vi "Position_TOTAL_R13.vi"(5 "Distance Between \nCameras  (*unit)":sgl=2.6) -> (0 "Valid Beacon Sets":bool[](array[boolean])=[TRUE, TRUE, TRUE, TRUE, TRUE], 12 "dX, dY\nLeft Cam":cluster{"X":sgl[], "Y":sgl[]}={"X"=[-3.0932024, -2.0237627, -0.92593014, 0.110565156, 1.1772758], "Y"=[9.218185, 9.218186, 9.218185, 9.218184, 9.218185]}, 13 "Position Valid":bool=TRUE, 14 "Left Camera Real Coordinates":cluster{"X":sgl, "Y":sgl}={"X"=9.218185, "Y"=3.507011}, 16 "dX, dY\nRight Cam":cluster{"X":sgl[], "Y":sgl[]}={"X"=[-5.4051104, -4.335671, -3.237838, -2.2013428, -1.1346322], "Y"=[8.902709, 8.902709, 8.902709, 8.902708, 8.902709]}, 17 "Distance to Each Beacon":cluster{" Right Cam":sgl[], " Left Cam":sgl[]}={" Right Cam"=[10.394308, 9.916446, 9.480992, 9.198957, 8.942072], " Left Cam"=[9.7002945, 9.453048, 9.272804, 9.247818, 9.26041]}, 18 "Robot Coordinates":cluster{"X":sgl, "Y":sgl}={"X"=9.060447, "Y"=4.662965}, 19 "Orietnation\n(current)":sgl=-7.7704344 format="%#_13g")   [LabVIEW 2015]
uses:
  <vilib>/Analysis/coordinate.llb/2D Cartesian Coordinate Rotation (Array).vi
  <vilib>/myRIO/Common/Instrument Driver Framework/myRIO v1.0/DIO/vis/myRIO v1.0 Close DIO.vi
  <vilib>/myRIO/Common/Instrument Driver Framework/myRIO v1.0/DIO/vis/myRIO v1.0 Unreserve DIO.vi
  <vilib>/myRIO/Common/Instrument Driver Framework/myRIO v1.0/DIO/vis/myRIO v1.0 Build MUX Configuration DIO.vi
  <vilib>/myRIO/Common/Instrument Driver Framework/myRIO v1.0/Resource Manager/vis/myRIO v1.0 Unreserve Channel List.vi
  <vilib>/myRIO/Common/Instrument Driver Framework/myRIO v1.0/Resource Manager/vis/myRIO v1.0 Create Configuration List.vi
  <vilib>/myRIO/Common/Instrument Driver Framework/myRIO v1.0/Resource Manager/vis/myRIO v1.0 Unreserve Channel.vi
  <vilib>/myRIO/Common/Instrument Driver Framework/myRIO v1.0/Resource Manager/vis/myRIO v1.0 Build Mutex Name.vi
  <vilib>/Instr/_visa.llb/VISA Configure Serial Port (Instr).vi
  <vilib>/myRIO/Common/Instrument Driver Framework/myRIO v1.0/DIO/vis/myRIO v1.0 Shutdown DIO.vi
  <vilib>/Utility/error.llb/Error Cluster From Error Code.vi
  <vilib>/myRIO/Common/Instrument Driver Framework/myRIO v1.0/Resource Manager/vis/myRIO v1.0 Configure IO.vi
  <vilib>/myRIO/Common/Instrument Driver Framework/Utilities/vis/Configuration Manager.vi
  <vilib>/myRIO/Common/Instrument Driver Framework/Utilities/vis/IO Manager.vi
  <vilib>/myRIO/Common/Instrument Driver Framework/myRIO v1.0/myRIO v1.0 Close.vi
  <vilib>/Analysis/NI_AALPro.lvlib
  <vilib>/myRIO/Instrument Drivers/Onboard IO/DIO/DIO.lvlib
panel:
  in  "Position Calc\nTimer":u32=50 caption="Position Calc Timer"
  in  "Max Dual\nBad Count":i32=10
  in  "Fetch Input\n(mSec)":u32=20 caption="Update Camera Input\n(mSec)"
  out "Right Data\nInput Flag\n- Internal":bool=TRUE
  in  "Position Calc\nReady":bool
  out "This Servo \nAngle - Right":sgl=88.125
  in  "Beacon Angles -R":sgl[](array[numeric])
  in  "Beacon Angles - L":sgl[](array[numeric])
  in  "Valid Angles -R":bool[](array[boolean])=[TRUE, TRUE, TRUE, TRUE, TRUE]
  in  "Valid Angles - L":bool[](array[boolean])=[TRUE, TRUE, TRUE, TRUE, TRUE]
  out "Left Data\nInput Flag\n- Internal":bool=TRUE
  in  "Check Shared Var Timer":u32=50 caption="Main Loop\n Timer (ms)"
  out "Left_Flag 2":bool
  out "Right_Flag 2":bool
  out "Beacons Found\n- Left (Bool Array) 2":bool[](array[boolean])=[TRUE, TRUE, TRUE, TRUE, TRUE]
  out "LEFT Beacon Coord - X px (IN) 2":sgl[](array[numeric])=[180.1461, 249.37689, 322.34314, 385.45602, 466.0847]
  out "LEFT Beacon Position - Y px (IN) 2":sgl[](array[numeric])=[301.75427, 303.58112, 297.41064, 306.23984, 296.68478]
  out "This Servo \nAngle - Left":sgl=88.125
  out "dT - Logic Loop":u32=134
  in  "Compliance Slope":u8=128
  in  "Max Search\n- Reactive Search Timeout":i32=10
  in  "Max Smart \nSearch Attempts":i32=50
  out "Search Count - R":u16
  out "Last Known\nTracking Position - R":u16=352
  out "Recovery Search Count R":i32
  out "Current Step - R":i8=9
  out "Response\nInduced - R":bool
  out "Response\nInduced - L":bool
  out "Pll Induced":bool
  out "Recovery Search Count L":i32
  out "deltaMoveServo\n- R":i16=52
  out "Move Respond - R":bool
  out "Move Respond - L":bool
  in  "Middle Beacon Coordinates":cluster{"X":sgl, "Y":sgl}={"X"=0.0, "Y"=2.5}
  out "Last Position":cluster{"X":sgl, "Y":sgl}
  out "Last Orientation":sgl
  in  "Distance\nBetween Beacons \n- Tolerance":sgl=0.35 format="%#_13g"
  in  "Distance\nBetween Beacons":sgl=1.0 format="%#_13g"
  out "atan2(y,x)":sgl
  out "dT":dbl
  in  "Orientation (-2) \nWeight":sgl=0.083333336 format="%#_13g"
  in  "Orientation (-1) \nWeight":sgl=0.16666667 format="%#_13g"
  in  "New Orientation \nThreshold":sgl=10.0
  out "Position Valid\nHistory":bool[](array[boolean])
  out "Orientation\nHistory":sgl[](array[numeric])
  out "Robot Coordinates\nHistory":cluster{sgl, sgl}[](array[cluster])
  in  "New Position \nThreshold":sgl=1.0
  in  "position(-2) weight":sgl=0.15 format="%#_13g"
  in  "position(-1) weight":sgl=0.35 format="%#_13g"
  out "Orientation Avgd":sgl
  in  "History Size":u8=10
  in  "Max Y (arena)":sgl=15.0
  in  "Max X (arena)":sgl=28.0
  in  "New Position\nWeight":sgl=0.5 format="%#_13g"
  in  "New Orientation\nWeight":sgl=0.75 format="%#_13g"
  in  "Max Std Dev (3)":sgl=0.2 format="%#_13g"
  in  "Max Std Dev (4)":sgl=0.2 format="%#_13g"
  out "Post Filtering\n- Valid Beacons":bool[](array[boolean])
  in  "New Pos\nThreshold (*unit)\nfilterd UNUSED":sgl=0.2
  out "Robot Coordinates - Avgd":cluster{"X":sgl, "Y":sgl}={"X"=9.06069, "Y"=4.637566}
  out "Real Position in Course 2":cluster{"X":dbl[], "Y":dbl[]}(graph)={"X"=[0.0, 0.0, 0.0, 0.0, 0.0, 9.060689926147461], "Y"=[0.5, 1.54, 2.58, 3.58, 4.58, 4.637566089630127]}
  out "Position \nLock Status":bool=TRUE
  in  "Max delta Angle":i32=1000
  out "Array 2":i16[](array[numeric])=[6, 1, 2, 14, 12]
  out "Right Camera Real Coordinate":cluster{"X":sgl, "Y":sgl}={"X"=8.902709, "Y"=5.8189187}
  in  "Start Search\nThreshold\n (x Wait Thres)":i32=5
  in  "Right Manual\nAngle":sgl=90.0
  in  "Left Manual\nAngle":sgl=90.0
  in  "MANUAL SERVO \nCONTROL ENABLE":bool
  out "deltaMoveServo\n- L":i16=52
  out "Last Known\nTracking Position - L":u16=352
  out "Search Count - L":u16
  in  "Search Step Size\n(deg)":sgl=10.0 format="%#_13g"
  out "Beacons Found\n- Right (Bool Array)":bool[](array[boolean])=[TRUE, TRUE, TRUE, TRUE, TRUE]
  out "RIGHT Beacon Position - Y px (IN)":sgl[](array[numeric])=[286.47595, 290.1055, 289.42014, 306.0349, 296.24573]
  out "RIGHT Beacon Coord - X px (IN)":sgl[](array[numeric])=[198.15767, 257.3629, 323.06607, 420.0157, 463.01376]
  in  "Right Servo\nID":string="\u0001"
  in  "Servo Comm\nWait Time - (ms)":i32
  in  "Left Servo\nID":string="\u0000"
  out "dT - Comm Loop":u32=134
  in  "Servo Comm\nLoop Time (ms)":i32=10
  in  "close comms":bool
  in  "Max Read\nTx Attempts":u8=3
  in  "Max Write\nTx Attempts":u8=3
  out "Current R (10bit)":u16=709
  out "Servo Moving - R":bool
  out "Servo Moving - L":bool
  out "Current L (10bit)":u16=352
  in  "SERVO ENABLE":bool=TRUE
  out "Move Servo - L":bool
  out "Move Servo - R":bool
  in  "Servo Goal Position\n - Right":u16=707
  in  "Move Servo\nThreshold (deg)":sgl=2.0 format="%#_13g"
  out "Current Step - L":i8=9
  in  "Angles Valid - L":bool=TRUE
  out "Wait Cycle Count - L":i32
  out "Wait Count - R":i32
  in  "Angles Valid - R":bool=TRUE
  in  "Wait Count\nFactor":i32=15
  in  "Servo Algorithm\nCycle Time(ms)":i32=50
  out "Direction - L":bool
  out "Direction - R":bool=TRUE
  in  "Servo Goal Position\n - Left":u16=353
  in  "Middle Beacon\nAngle - Left":sgl=87.88366
  in  "Current Angle\n - Left (internal)":sgl=88.125
  in  "Middle Beacon\nAngle - Right":sgl=102.09343
  in  "Current Angle\n - Right (internal)":sgl=102.71484
  in  "stop":bool
  in  "Num of Beacons (Total)":i8=5
  out "Angle to Pixel Ratios":T1={"Angle to Pixel\nRatio - Horizontal"=0.090625, "Angle to Pixel\nRatio - Vertical"=0.09375} {"Angle to Pixel\nRatio - Vertical" format="%#_13g"; "Angle to Pixel\nRatio - Horizontal" format="%#_13g"}
  in  "Cam AOV Vertical (deg)":sgl=45.0
  in  "Cam AOV Horizontal (deg)":sgl=58.0
  in  "Image Height (px)":sgl=480.0
  in  "Image Width (px)":sgl=640.0
  out "Beacon Coordinates - Left Image":T2={"Beacon Position - X px"=[-75.0, 0.0, 102.0], "Beacon Position - Y px"=[133.0, 0.0, 40.0]}
  out "Beacon Coordinates - Right Image":T2
  out "Distance to LBF":sgl[](array[numeric])=[0.024284193, 0.015691843, 0.008273765, 0.028971607, 0.03291407]
  out "Local Coordinates - Calculated":cluster{sgl[], sgl[]}(graph)={[-1.8217448, -0.75672, 0.3300292, 1.3598052, 2.408354], [9.527695, 9.422711, 9.26693, 9.147298, 8.941757]}
  out "Local Coordinates - Adjusted":cluster{sgl[], sgl[]}(graph)={[-1.8184614, -0.75884163, 0.32891047, 1.3558882, 2.4128041], [9.551756, 9.407164, 9.258732, 9.118592, 8.974369]}
  out "Normalized Beacons\nCoordinates Relative\nto Robot\n- Local":cluster{"X":sgl[], "Y":sgl[]}={"X"=[-1.8184614, -0.75884163, 0.32891047, 1.3558882, 2.4128041], "Y"=[9.551756, 9.407164, 9.258732, 9.118592, 8.974369]}
  out "Local Coordinates - Rotated":cluster{dbl[], dbl[]}(graph)={[2.311907982053154, -3.093202399055953, -2.02376281856378, -0.9259301209089894, 0.11056515513330578, 1.1772757583589313], [0.3154767124369396, 9.218185381048452, 9.218185941536527, 9.218185875284743, 9.218184915244796, 9.218185579154817]}
  out "All Object Coordinates \n- Local - Rotated":cluster{"X":sgl[], "Y":sgl[]}={"X"=[2.311908, -3.0932024, -2.0237627, -0.92593014, 0.110565156, 1.1772758], "Y"=[0.31547672, 9.218185, 9.218186, 9.218185, 9.218184, 9.218185]}
  out "Local Coordinates - Normalized":cluster{sgl[], dbl[]}(graph)={[2.3333333, -1.8184614, -0.75884163, 0.32891047, 1.3558882, 2.4128041], [0.0, 9.551755905151367, 9.407163619995117, 9.258731842041016, 9.118592262268066, 8.974369049072266]}
  in  "Max Std Dev (5)":sgl=0.2 format="%#_13g"
  out "All Object Coordinates \n- Local":cluster{"X":sgl[], "Y":sgl[]}={"X"=[2.3333333, -1.8184614, -0.75884163, 0.32891047, 1.3558882, 2.4128041], "Y"=[0.0, 9.551756, 9.407164, 9.258732, 9.118592, 8.974369]}
  out "LOCAL\nBeacon Coordinates\nRelative to Robot":cluster{"dX_beacon":sgl[], "dY_beacon":sgl[]}={"dX_beacon"=[-1.8217448, -0.75672, 0.3300292, 1.3598052, 2.408354], "dY_beacon"=[9.527695, 9.422711, 9.26693, 9.147298, 8.941757]}
  out "dA2":sgl=15.074211 format="%#_13g"
  out "All Same\nDirection":bool=TRUE
  out "Valid Data\nSets":bool[](array[boolean])=[TRUE, TRUE, TRUE, TRUE, TRUE]
  in  "Distance Threshold\nRef Triangles (*unit)":sgl=20.0
  in  "Real Beacon\n - Coordinates":cluster{"X":dbl[], "Y":dbl[]}={"X"=[0.0, 0.0, 0.0, 0.0, 0.0, 0.0], "Y"=[0.5, 1.5, 2.5, 3.5, 4.5, 0.0]}
  # "POSITION CALCULATION VARIABLES"
  # "OUTPUT VALUES"
  # "CONFIG VALUES"
  # "FILTER CONFIG VALUES"
  # "FEEDBACK INPUT VALUES"
  # "INPUT VALUES"
  # "INTERMEDIATE VALUES"
  # "IMAGE TO ANGLE VARIABLES"
  # "VISION PROCESSEING INPUTS"
  # "Use moving average for previous orientation thresholds"
  # "INPUTS"
  # "CONFIG"
  # "OUTPUT VALUES"
  # "*********************"
  # "unfiltered"
  # "NEW FILTER VALS"
  # "Inter Beacon Distance Filtering"
  # "SERVO CONTROL VARIABLES"
  # "SERVO CONTROL VARIABLES"
  # "CONFIG"
  # "SHARED VARIABLE INPUTS"
  # "LOCAL VARIABLE INPUTS"
  # "INTERNRAL VARIABLES"
  # "SEARCH ROUTINE VARIABLES"
  # "MISC"
  # "SERVO IDs"
  # "CONTROL DELAYS"
  # "COMM LOOP DELAY"
  # "COMM PROTOCOL"
  # "1 Search Cycle is Certain\nNumber of Wait Cycles"
  # "Servo Enable must be false**"
  # "Make function of distance^^"
  # "**** only left side starts search\nat previously known good angle"
  # "change to only use\nthis max delta angle\nwhen enabled"
  # "NOTE: Must be 1 bigger than amount of beacons"
  # "NOTE: Must be 1 bigger than amount of beacons"
types:
  T1 = cluster{"Angle to Pixel\nRatio - Horizontal":sgl, "Angle to Pixel\nRatio - Vertical":sgl}
  T2 = cluster{"Beacon Position - X px":sgl[], "Beacon Position - Y px":sgl[]}
  T3 = cluster{"Array of Double":dbl[], "Array of Double":dbl[]}
  T4 = typedef "DIO.lvlib/DIO Reference.ctl" = cluster{"myRIO Reference":T5, "DIO Channels List":T9}
  T5 = typedef "myRIO Generic Hardware Reference.ctl" = cluster{"myRIO Model":T6, "myRIO Hardware Reference":T7}
  T6 = typedef "Hardware Version Enum.ctl" = enum16{"Unknown", "myRIO-1900", "myRIO-1950", "roboRIO"}
  T7 = typedef "myRIO v1.0 Reference.ctl" = cluster{"Generic FPGA Reference":T8, "Allow multiple opens":bool}
  T8 = typedef "Generic FPGA Reference.ctl" = refnum<k20>
  T9 = typedef "DIO Channels List.ctl" = T10[]
  T10 = typedef "DIO Channels Enum.ctl" = enum16{"Not Connected", "C/DIO0", "C/DIO1", "C/DIO2", "C/DIO3", "C/DIO4", "C/DIO5", "C/DIO6", "C/DIO7", "A/DIO0", "A/DIO1", "A/DIO2", "A/DIO3", "A/DIO4", "A/DIO5", "A/DIO6", "A/DIO7", "A/DIO8", "A/DIO9", "A/DIO10", "A/DIO11", "A/DIO12", "A/DIO13", "A/DIO14", "A/DIO15", "B/DIO0", "B/DIO1", "B/DIO2", "B/DIO3", "B/DIO4", "B/DIO5", "B/DIO6", "B/DIO7", "B/DIO8", "B/DIO9", "B/DIO10", "B/DIO11", "B/DIO12", "B/DIO13", "B/DIO14", "B/DIO15", "LED0", "LED1", "LED2", "LED3", "Button0", "DIO/DIO0", "DIO/DIO1", "DIO/DIO2", "DIO/DIO3", "DIO/DIO4", "DIO/DIO5", "DIO/DIO6", "DIO/DIO7", "DIO/DIO8", "DIO/DIO9", "SPI/CS0", "SPI/CS1", "SPI/CS2", "SPI/CS3", "LED RADIO (Green)", "LED RADIO (Red)", "LED COMM (Green)", "LED COMM (Red)", "LED MODE (Green)", "LED MODE (Red)"}
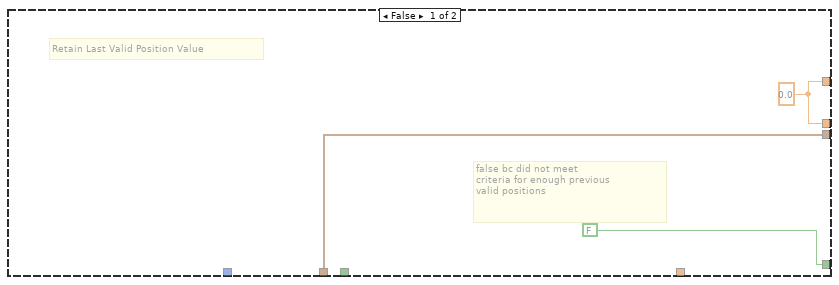
[diagram p6: hidden frame]
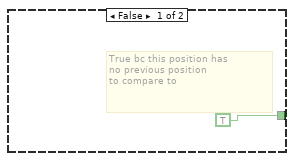
[diagram p7: hidden frame]
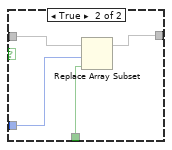
[diagram p9: hidden frame]
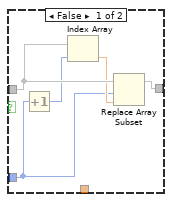
[diagram p10: hidden frame]
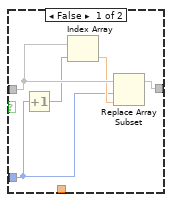
[diagram p11: hidden frame]
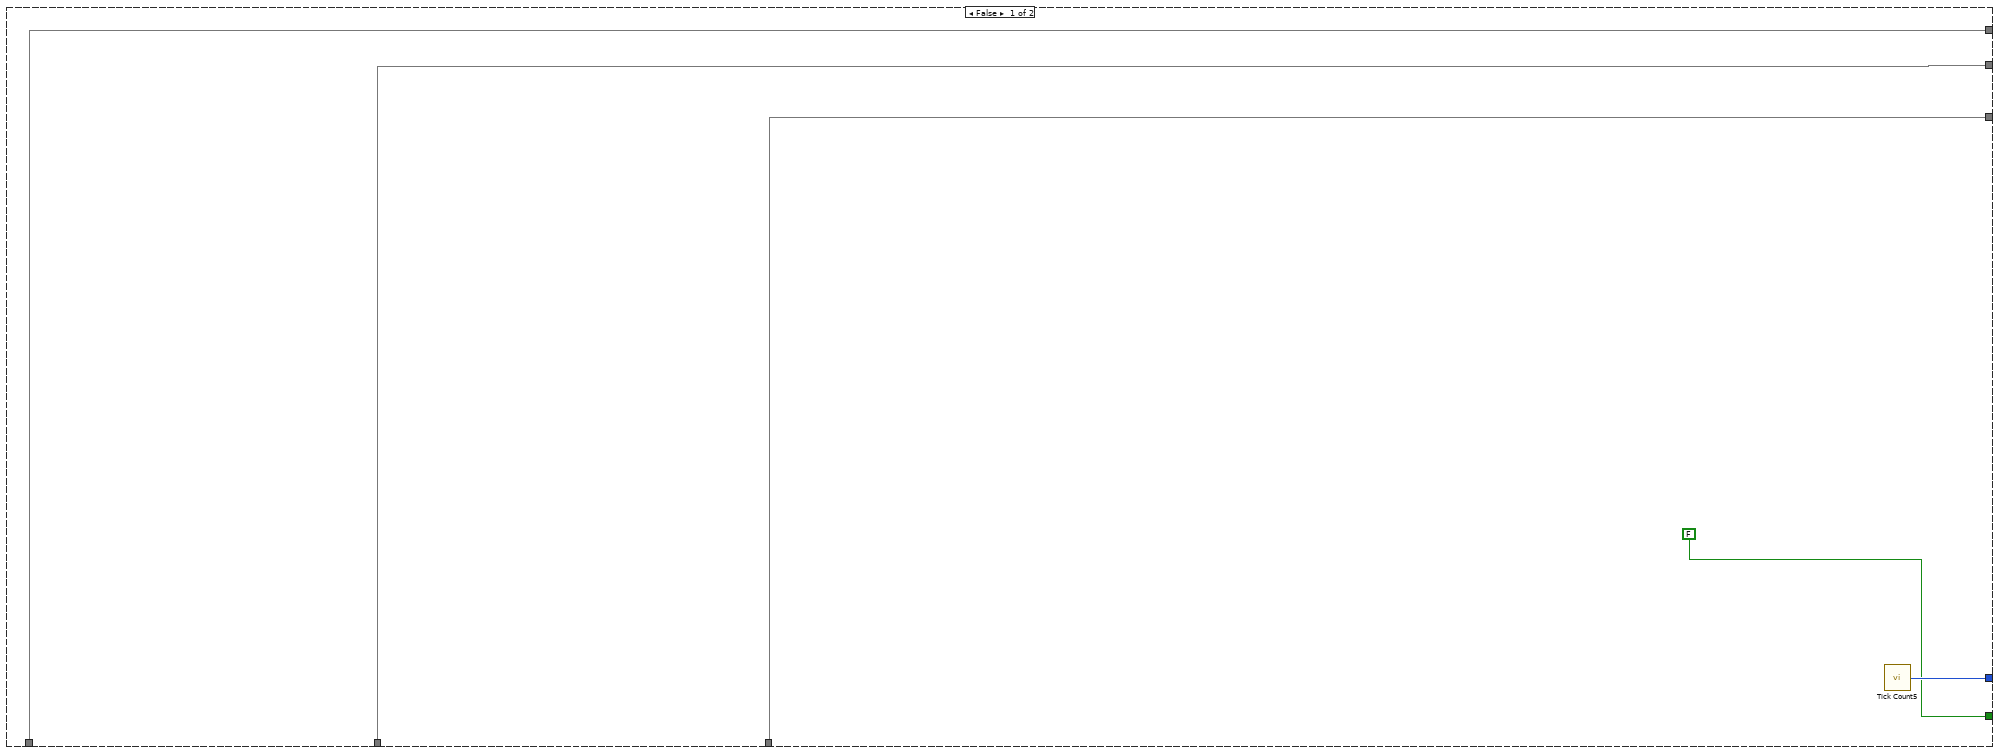
[diagram p14: hidden frame]
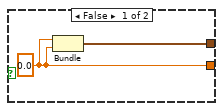
[diagram p16: hidden frame]
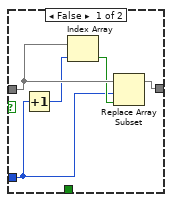
[diagram p17: hidden frame]
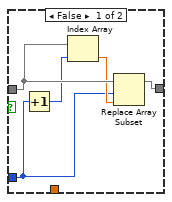
[diagram p18: hidden frame]
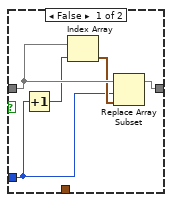
[diagram p19: hidden frame]
diagram:
  w4 = FALSE
  w1 = FALSE
  w23 = sgl 0.0
  w15 = u16 35
  w16 = u16 512
  # "Completel Search Mode"
  # "Read Inputs when Available"
  # "# of Physical Beacons"
  # "Right Data Internal Falg"
  # "Left Data Internal Falg"
  # "Start at (or around)\nMax Smart Search\nso system will\nimmediately begin to search"
  # "Recovery Search -5"
  # "Recovery Search - L"
  # "Search Count - R"
  # "Direction - R"
  # "Direction - L"
  # "Wait Cycle Count"
  # "Search Cycle Count - R"
  # "Last Known Track\nAngle - R"
  # "Move Respond - R"
  # "Move Respond - L"
  # "Move Respond - R"
  # "Move Respond - L"
  # "Wait Cycle Count"
  # "Last Known Track\nAngle"
  # "Search Count - L"
  # "delta Move Angle - R\n(Sum)"
  # "delta Move Angle - L\n(Sum)"
  # "delta Move Angle - R"
  # "delta Move Angle - L"
  # "Last Known Track\nAngle - L"
  # "Initialize Shift Arrays"
  # "Robot Position (cluster)\nShift Array"
  # "Robot Position (cluster)\nShift Array"
  # "Position Valid Shift Array"
  # "Orientation Shift Array"
  # "Position Valid Shift Array"
  # "Orientation Shift Array"
  # "***********************************"
  # "Search Cycle Count - L"
  # "Servo Communication (to Servo- UART))"
  # "Wait Cycle Counter - R"
  # "Internal Local Variables"
  # "Servo Control Logic"
  # "Wait Cycle Counter - L"
  # "Local Variables"
  # "Images to Robot Position Calculation Process"
  # "SERVO MOTOR CONTROL"
  # "SERVO MOTOR CONTROL"
  n1 = Divide(x="Cam AOV Horizontal (deg)", y="Image Width (px)") -> (x/y=w9:sgl)
  n2 = Divide(x="Cam AOV Vertical (deg)", y="Image Height (px)") -> (x/y=w10:sgl)
  n3 = Bundle(w9, w10) -> (w3:cluster{sgl, sgl})  [unwired: 1 in]
  "Angle to Pixel Ratios" <- w3
  n4 = disable-structure shown="Disabled" {
    frame Disabled {
      # "Always Read Incoming Flags & Store"
      n5 = while {
        tunnel: "Check Shared Var Timer" -> [w40]
        stop <- FALSE stop-if-true
        n6 = shared-variable "myRIO-1900\\Lib1.lvlib\\RIGHT_FLAG"() -> (→"Right_Flag 2":bool)  [unwired: 1 in, 1 out]
        n7 = shared-variable "myRIO-1900\\Lib1.lvlib\\Left_Flag"() -> (→"Left_Flag 2":bool)  [unwired: 1 in, 1 out]
        n8 = call "Wait8"("Count(mSec)"=w40) -> ()  [unwired: 1 out]
      }
    }
    frame Enabled {
    }
  }
  n9 = while {
    shift-right: [w48] -> _
    shift-left: w4 -> [w54]
    shift-right: [w47] -> _
    shift-left: w4 -> [w52]
    tunnel: w3 -> [w50]
    tunnel: "Num of Beacons (Total)" -> [w51]
    stop <- FALSE stop-if-true
    # "Wait for Both Internal Flags"
    n10 = call "Wait6"("Count(mSec)"="Fetch Input\n(mSec)") -> ()  [unwired: 1 out]
    n11 = shared-variable "RT myRIO Target - Overlord\\Localization_Variables_r0.lvlib\\RIGHT_FLAG"() -> (w44:bool)  [unwired: 1 in, 1 out]
    n12 = shared-variable "RT myRIO Target - Overlord\\Localization_Variables_r0.lvlib\\Left_Flag"() -> (w45:bool)  [unwired: 1 in, 1 out]
    n13 = case shown="True" w44 {
      tunnel: w51 -> [_ w68]
      tunnel: w50 -> [_ w66]
      tunnel: [w55 TRUE] -> w43
      tunnel: w52 -> [w55 _]
      frame False {
        # "Don't Update Servo Position\nbc we're waiting on new Data to\ncome in and the servo position\nwas set at the previous set of data"
      }
      frame True {
        # "Store Values"
        # "Raise Internal Flag"
        # "If New Data Available"
        # "From Shift Reg"
        # "Perforrm Indivudual Angle Calculation"
        # "Pull Down Individual Flag"
        n14 = shared-variable "RT myRIO Target - Overlord\\Localization_Variables_r0.lvlib\\RIGHT_BEACON_X_array"() -> (w60:dbl[])  [unwired: 1 in, 1 out]
        "RIGHT Beacon Coord - X px (IN)" <- w60
        n15 = shared-variable "RT myRIO Target - Overlord\\Localization_Variables_r0.lvlib\\RIGHT_BEACON_Y_array"() -> (w59:dbl[])  [unwired: 1 in, 1 out]
        "RIGHT Beacon Position - Y px (IN)" <- w59
        n16 = shared-variable "RT myRIO Target - Overlord\\Localization_Variables_r0.lvlib\\RIGHT_BEACON_BOOL_array"() -> (w58:bool[])  [unwired: 1 in, 1 out]
        "Beacons Found\n- Right (Bool Array)" <- w58
        n17 = Bundle("Array of Double"=w60, "Array of Double"=w59) -> (w57:T3)  [unwired: 1 in]
        "Beacon Coordinates - Right Image" <- w57
        n18 = shared-variable "RT myRIO Target - Overlord\\Localization_Variables_r0.lvlib\\Right Servo Angle_Image"() -> (w56:dbl)  [unwired: 1 in, 1 out]
        "This Servo \nAngle - Right" <- w56
        n19 = shared-variable "RT myRIO Target - Overlord\\Localization_Variables_r0.lvlib\\RIGHT_FLAG"(FALSE) -> ()  [unwired: 1 in, 1 out]
        n20 = feedback #1() -> (w70:sgl[])  [unwired: 1 in]
        n21 = feedback #2() -> (w69:bool[])  [unwired: 1 in]
        n22 = call "Angle Calc_Individual Process R2.vi"("Angle to Pixel Ratios"=w66, "Previous Angles"=w70, "Num of Beacons"=w68, "Beacon Coordinates - Image"=w57, "Current Servo Angle"=w56, "Beacons Found (Bool Array)"=w58, "Previous Valid Angles"=w69) -> ("Servo Goal Angle"=w65:dbl, "Valid Beacons (Bool Array)\nPosition Calc"=w63:bool[], "Angle Of Beacons \nRelative to Robot"=w62:sgl[], "Angles Valid\nServo Control"=w64:bool)  [unwired: 2 in, 3 out]
        n23 = feedback-in #1(w62) -> ()
        n24 = feedback-in #2(w63) -> ()
        n25 = local write "Middle Beacon\nAngle - Right"(w65) -> ()
        n26 = local write "Angles Valid - R"(w64) -> ()
        n27 = local write "Beacon Angles -R"(w62) -> ()
        n28 = local write "Valid Angles -R"(w63) -> ()
      }
    }
    "Right Data\nInput Flag\n- Internal" <- w43
    n29 = case shown="True" w45 {
      tunnel: [w71 TRUE] -> w49
      tunnel: w54 -> [w71 _]
      tunnel: w50 -> [_ w74]
      tunnel: w51 -> [_ w73]
      frame False {
        # "Don't Update Servo Position\nbc we're waiting on new Data to\ncome in and the servo position\nwas set at the previous set of data"
      }
      frame True {
        # "Store Values"
        # "Raise Internal Flag"
        # "If New Data Available"
        # "Perforrm Indivudual Angle Calculation"
        # "Pull Down Individual Flag"
        n30 = shared-variable "RT myRIO Target - Overlord\\Localization_Variables_r0.lvlib\\LEFT_BEACON_X_array"() -> (w82:dbl[])  [unwired: 1 in, 1 out]
        "LEFT Beacon Coord - X px (IN) 2" <- w82
        n31 = shared-variable "RT myRIO Target - Overlord\\Localization_Variables_r0.lvlib\\LEFT_BEACON_Y_array"() -> (w83:dbl[])  [unwired: 1 in, 1 out]
        "LEFT Beacon Position - Y px (IN) 2" <- w83
        n32 = shared-variable "RT myRIO Target - Overlord\\Localization_Variables_r0.lvlib\\LEFT_BEACON_BOOL_array"() -> (w84:bool[])  [unwired: 1 in, 1 out]
        "Beacons Found\n- Left (Bool Array) 2" <- w84
        n33 = Bundle("Array of Double"=w82, "Array of Double"=w83) -> (w80:T3)  [unwired: 1 in]
        "Beacon Coordinates - Left Image" <- w80
        n34 = shared-variable "RT myRIO Target - Overlord\\Localization_Variables_r0.lvlib\\Left Servo Angle_Image"() -> (w72:dbl)  [unwired: 1 in, 1 out]
        "This Servo \nAngle - Left" <- w72
        n35 = shared-variable "RT myRIO Target - Overlord\\Localization_Variables_r0.lvlib\\Left_Flag"(FALSE) -> ()  [unwired: 1 in, 1 out]
        n36 = feedback #3() -> (w86:sgl[])  [unwired: 1 in]
        n37 = feedback #4() -> (w85:bool[])  [unwired: 1 in]
        n38 = call "Angle Calc_Individual Process R2.vi"("Angle to Pixel Ratios"=w74, "Previous Angles"=w86, "Num of Beacons"=w73, "Beacon Coordinates - Image"=w80, "Current Servo Angle"=w72, "Beacons Found (Bool Array)"=w84, "Previous Valid Angles"=w85) -> ("Servo Goal Angle"=w79:dbl, "Valid Beacons (Bool Array)\nPosition Calc"=w77:bool[], "Angle Of Beacons \nRelative to Robot"=w76:sgl[], "Angles Valid\nServo Control"=w78:bool)  [unwired: 2 in, 3 out]
        n39 = feedback-in #3(w76) -> ()
        n40 = feedback-in #4(w77) -> ()
        n41 = local write "Middle Beacon\nAngle - Left"(w79) -> ()
        n42 = local write "Beacon Angles - L"(w76) -> ()
        n43 = local write "Angles Valid - L"(w78) -> ()
        n44 = local write "Valid Angles - L"(w77) -> ()
      }
    }
    "Left Data\nInput Flag\n- Internal" <- w49
    n45 = And(x=w49, y=w43) -> (x .and. y?=w53:bool)
    n46 = case shown="True" w53 {
      selector: w53 -> [_ w89]
      tunnel: w49 -> [w88 _]
      tunnel: [w88 w90] -> w48
      tunnel: [w87 w90] -> w47
      tunnel: w43 -> [w87 _]
      frame False {
      }
      frame True {
        w90 = FALSE
        # "Reset Internal Data Flags"
        # "Position Data\nReady Enabled"
        n47 = local write "Position Calc\nReady"(w89) -> ()
      }
    }
  }
  n48 = Bundle(w23, w23) -> (w26:cluster{sgl, sgl})  [unwired: 1 in]
  n49 = Initialize Array(w23, "History Size") -> (w21:sgl[])
  n50 = Initialize Array(w26, "History Size") -> (w22:cluster{sgl, sgl}[])
  n51 = Initialize Array(FALSE, "History Size") -> (w20:bool[])
  n52 = call "Tick Count4"() -> ("Tick Count(uSec)"=w19:u32)
  n53 = while {
    shift-right: [w101] -> _
    shift-left: w21 -> [w98]
    shift-right: [w100] -> _
    shift-left: w20 -> [w99]
    shift-right: [w102] -> _
    shift-left: w22 -> [w93]
    shift-right: [w94] -> _
    shift-left: w19 -> [w95]
    stop <- "stop" stop-if-true
    n54 = call "Wait5"("Count(mSec)"="Position Calc\nTimer") -> ()  [unwired: 1 out]
    n55 = case shown="True" "Position Calc\nReady" {
      selector: "Position Calc\nReady" -> [_ w114]
      tunnel: w93 -> [_ w151]
      tunnel: w93 -> [w111 w141]
      tunnel: w98 -> [w113 w140]
      tunnel: w99 -> [w112 w139]
      tunnel: [w113 w138] -> w101
      tunnel: [w112 w133] -> w100
      tunnel: [w111 w137] -> w102
      tunnel: w99 -> [_ w136]
      tunnel: w98 -> [_ w135]
      tunnel: [w110 w126] -> w96
      tunnel: w95 -> [_ w126]
      tunnel: [FALSE TRUE] -> w97
      tunnel: w93 -> [_ w121]
      frame False {
        n56 = call "Tick Count5"() -> ("Tick Count(uSec)"=w110:u32)
      }
      frame True {
        # "Update Outputs\nif Current Calc is Invalid\n(shouldn't matter)"
        # "Estimate Orienation Based on Previous Position"
        # "****# of previous in history that must be true\nin order for position to be considered \"locked\""
        # "New Position is Valid if both \nOrientation and Positions\nis within range of previous"
        # "Robot Position\n Shift Array"
        # "Position Valid Shift Array"
        # "Orientation Shift Array"
        # "Orientation Value"
        # "Shift & Insert Current Position Valid"
        # "Position Valid\n(orientation)"
        # "Position Valid\n(position)"
        # "Update Shift Registers"
        # "Shift & Insert Current Calculated Orientation"
        # "Shift & Insert Current Robot Position"
        # "UPDATE FINAL OUTPUT\n VALUES"
        # "Find Common Beacons\nAmong Cameras"
        # "Valid Beacon Sets"
        # "Currently will only\ncalculate position if 2+ \nbeacons are available \nfrom both cameras"
        n57 = Not(x=w114) -> (.not. x?=w115:bool)
        n58 = local write "Position Calc\nReady"(w115) -> ()
        n59 = disable-structure shown="Disabled" {
          disable-tunnel: "Valid Angles - L" -> [w216 _]
          disable-tunnel: "Valid Angles -R" -> [w215 _]
          frame Disabled {
            # "Each has at \nleast 1 beacon"
            n60 = Boolean Array To Number(Boolean array=w215) -> (number=w217:u32)
            n61 = Boolean Array To Number(Boolean array=w216) -> (number=w218:u32)
            n62 = Greater Than 0?(x=w217) -> (x > 0?=w219:bool)
            n63 = Greater Than 0?(x=w218) -> (x > 0?=w220:bool)
            n64 = And(x=w220, y=w219) -> ()  [unwired: 1 out]
          }
          frame Enabled {
          }
        }
        n65 = And(x="Valid Angles - L", y="Valid Angles -R") -> (x .and. y?=w152:bool[])
        "Valid Beacon Sets" <- w152
        n66 = local read "Num of Beacons (Total)"() -> (w116:i8)
        n67 = Boolean To (0,1)(Boolean=w152) -> (0, 1=w156:i16[])
        n68 = Add Array Elements(numeric array=w156) -> (sum=w155:i16)
        n69 = Greater?(x=w155, y=1) -> (0:w153:bool)
        n70 = case shown="True" w153 {
          tunnel: w152 -> [_ w237]
          tunnel: "Beacon Angles - L" -> [_ w235]
          tunnel: "Beacon Angles -R" -> [_ w234]
          tunnel: w116 -> [_ w236]
          tunnel: w152 -> [_ w232]
          tunnel: w151 -> [_ w231]
          tunnel: [w222 w230] -> w143
          tunnel: [w223 w229] -> w124
          tunnel: [w223 w228] -> w123
          tunnel: [w221 w227] -> w144
          tunnel: w136 -> [_ w226]
          tunnel: w135 -> [_ w225]
          tunnel: w121 -> [_ w224]
          frame False {
            w221 = sgl 0.0 ("f")
            w223 = FALSE
            # "FALSE"
            # "F"
            n71 = Bundle("f"=w221, "f"=w221) -> (w222:cluster{"f":sgl, "f":sgl})  [unwired: 1 in]
          }
          frame True {
            # "Number of Beacons"
            # "**maybe add case\nto handle if some arent\nsame direction"
            # "Check 1st element\nwith rest of elements"
            # "Find delta X and delta Y\nto Each Camera from Each Beacon"
            # "Make Sure all Pointed \nIn Same Direction"
            # "For Each Valid Beacon\nCalculate Distance from Each Camera to Each Beacon"
            n72 = for {
              N: w236 -> [_]
              tunnel: w237 -> [w711] mode=indexing
              tunnel: w235 -> [w710] mode=indexing
              tunnel: w234 -> [w709] mode=indexing
              tunnel: "Distance Between \nCameras  (*unit)" -> [w708]
              tunnel: "Distance Threshold\nRef Triangles (*unit)" -> [w707]
              tunnel: [w706] -> w242 mode=indexing
              tunnel: [w705] -> _ mode=indexing
              tunnel: [w704] -> w243 mode=indexing
              tunnel: [w703] -> w239 mode=indexing
              tunnel: [w702] -> w238 mode=indexing
              tunnel: [w701] -> w244 mode=indexing
              n73 = case shown="True" w711 {
                tunnel: w710 -> [w716 w726]
                tunnel: w709 -> [w715 w725]
                tunnel: w708 -> [_ w717]
                tunnel: w707 -> [_ w718]
                tunnel: [w716 w724] -> w706
                tunnel: [w715 w723] -> w705
                tunnel: [FALSE w722] -> w704
                tunnel: [w713 w721] -> w703
                tunnel: [w713 w720] -> w702
                tunnel: [0 w719] -> w701
                frame False {
                  w713 = sgl 1.0
                }
                frame True {
                  # "Build Reference Triangle"
                  n74 = call "Position Calc_Build Reference Triangle_R1.vi"("A2_in"=w726, "A3_in"=w725, "S1 (Length Between\n Cameras - inches)"=w717, "Distance\nThreshold"=w718) -> ("S2"=w721:sgl, "S3"=w720:sgl, "Direction"=w719:i8, "A2"=w724:sgl, "A3"=w723:sgl, "Accept"=w722:bool)  [unwired: 6 in]
                }
              }
            }
            "Valid Data\nSets" <- w243
            n75 = Bundle(w239, w238) -> (→"Distance to Each Beacon":cluster{sgl[], sgl[]})  [unwired: 1 in]
            n76 = Boolean To (0,1)(Boolean=w243) -> (0, 1=w252:i16[])
            n77 = for {
              N: w236 -> [_]
              tunnel: w243 -> [w254] mode=indexing
              tunnel: w244 -> [w255] mode=indexing
              tunnel: [w255] -> w249 mode=indexing if=w254
              # "Only add to array\nif valid distance"
            }
            n78 = Add Array Elements(numeric array=w252) -> (sum=w240:i16)
            n79 = Greater?(x=w240, y=1) -> (0:w246:bool)
            n80 = Index Array(array=w249, index=0) -> (element=w248:i32)
            n81 = Equal?(x=w249, y=w248) -> (x = y?=w247:bool[])
            n82 = And Array Elements(Boolean array=w247) -> (logical AND=w245:bool)
            "All Same\nDirection" <- w245
            n83 = case shown="True" w245 {
              tunnel: w236 -> [_ w276]
              tunnel: w243 -> [_ w280]
              tunnel: w246 -> [_ w279]
              tunnel: w238 -> [_ w277]
              tunnel: w239 -> [_ _]
              tunnel: w242 -> [_ w278]
              tunnel: w240 -> [_ w275]
              tunnel: w239 -> [_ w274]
              tunnel: w238 -> [_ w273]
              tunnel: w235 -> [_ w272]
              tunnel: w234 -> [_ w271]
              tunnel: w232 -> [_ w270]
              tunnel: "Distance Between \nCameras  (*unit)" -> [_ w269]
              tunnel: w231 -> [_ w268]
              tunnel: [w257 w267] -> w230
              tunnel: [w258 w266] -> w229
              tunnel: [w258 w265] -> w228
              tunnel: [w256 w264] -> w227
              tunnel: w226 -> [_ w263]
              tunnel: w225 -> [_ w262]
              tunnel: w224 -> [_ w261]
              frame False {
                w256 = sgl 0.0 ("f")
                w258 = FALSE
                w259 = 0
                w260 = sgl 0.0
                (unwired) FALSE
                # "FALSE"
                n84 = Build Array(w260, w260, w260) -> ()  [unwired: 1 out]
                n85 = Build Array(w260, w260, w260) -> ()  [unwired: 1 out]
                n86 = Build Array(w260, w260, w260) -> ()  [unwired: 1 out]
                n87 = Build Array(w260, w260, w260) -> ()  [unwired: 1 out]
                n88 = Build Array(w260, w260, w260) -> ()  [unwired: 1 out]
                n89 = Build Array(w260, w260, w260) -> ()  [unwired: 1 out]
                n90 = Build Array(w259, w259, w259) -> ()  [unwired: 1 out]
                n91 = Bundle("f"=w256, "f"=w256) -> (w257:cluster{"f":sgl, "f":sgl})  [unwired: 1 in]
              }
              frame True {
                # "All Values in Same Direction"
                n92 = case shown="True" w279 {
                  tunnel: w276 -> [_ w298]
                  tunnel: w280 -> [_ w368]
                  tunnel: w278 -> [_ w367]
                  tunnel: w277 -> [_ w366]
                  tunnel: w275 -> [_ _]
                  tunnel: w274 -> [_ _]
                  tunnel: w273 -> [_ _]
                  tunnel: w272 -> [_ _]
                  tunnel: w271 -> [_ _]
                  tunnel: w270 -> [_ _]
                  tunnel: w269 -> [_ w331]
                  tunnel: w268 -> [_ w316]
                  tunnel: [w283 w313] -> w267
                  tunnel: [w281 w310] -> w266
                  tunnel: [w281 w304] -> w265
                  tunnel: [w282 w301] -> w264
                  tunnel: w263 -> [_ w305]
                  tunnel: w262 -> [_ w306]
                  tunnel: w261 -> [_ w294]
                  frame False {
                    w282 = sgl 0.0 ("f")
                    w281 = FALSE
                    w284 = 0
                    w285 = sgl 0.0
                    (unwired) FALSE
                    # "FALSE"
                    # "1 Valid Data Set\n\nRun Single Position Calc for each?\n\nor estimate position based on previous \nposition and orientation"
                    n93 = Build Array(w285, w285, w285) -> ()  [unwired: 1 out]
                    n94 = Build Array(w285, w285, w285) -> ()  [unwired: 1 out]
                    n95 = Build Array(w285, w285, w285) -> ()  [unwired: 1 out]
                    n96 = Build Array(w285, w285, w285) -> ()  [unwired: 1 out]
                    n97 = Build Array(w285, w285, w285) -> ()  [unwired: 1 out]
                    n98 = Build Array(w285, w285, w285) -> ()  [unwired: 1 out]
                    n99 = Build Array(w284, w284, w284) -> ()  [unwired: 1 out]
                    n100 = Bundle("f"=w282, "f"=w282) -> (w283:cluster{"f":sgl, "f":sgl})  [unwired: 1 in]
                  }
                  frame True {
                    w342 = sgl 2.0
                    w361 = 0
                    # "Only Apply This Filtering \nif 3 or More Beacons Still Valid"
                    # "Orientation Value"
                    # "Orientation Valid"
                    # "Y (current)"
                    # "X (current)"
                    # "Number of Valid\nPrevious Orientations"
                    # "Position Valid Shift Array"
                    # "More than 1 Previous\nValid Positions"
                    # "More than\n1 previous position\navailable"
                    # "Choose Beacon Set\nwith Lowest Std Dev"
                    # "Y value cannot be negative"
                    # "Find New # Of Valid Beacons"
                    # "Adjust/Normalize\nLocal Beacon Positions\nusing Line of Best fit"
                    # "# Valid\nData Sets"
                    # "cam, y"
                    # "cam, x"
                    # "Calculate dX and dY\nfor right cam"
                    # "Average dX and dY from each (valid) beacon to find position of each camera\n\nthen average all  positions for each camera find center between"
                    # "Convert Slope\nto Radians"
                    # "*rotate CCW in rad"
                    # "Rotate Coordinate\n System by Slope"
                    # "2+ Data Sets"
                    n101 = for {
                      N: w298 -> [_]
                      tunnel: w368 -> [w669] mode=indexing
                      tunnel: w367 -> [w673] mode=indexing
                      tunnel: w366 -> [w672] mode=indexing
                      tunnel: [w671] -> w324 mode=indexing
                      tunnel: [w670] -> w323 mode=indexing
                      tunnel: [w668] -> w309 mode=indexing
                      n102 = case shown="True" w669 {
                        selector: w669 -> [w675 w679]
                        tunnel: w673 -> [_ w687]
                        tunnel: [w674 w677] -> w671
                        tunnel: [w674 w678] -> w670
                        tunnel: w672 -> [_ w676]
                        tunnel: [w675 w679] -> w668
                        frame False {
                          w674 = sgl 0.0
                          # "Current Data Set Was Not Valid\nFill with 0\nWill not be used later"
                        }
                        frame True {
                          # "dY"
                          # "dX"
                          # "Negate dX if A2>90"
                          # "Find LOCAL Coordinate of Each Beacon"
                          # "Current - Valid Data Set"
                          n103 = Less?(x=w687, y=sgl 90.0) -> (x < y?=w689:bool)
                          n104 = case shown="False" w689 {
                            tunnel: w687 -> [w696 w698]
                            tunnel: [w694 w699] -> w686
                            tunnel: [FALSE TRUE] -> w681
                            frame False {
                              # "Negative Y"
                              # "A2 is > 90"
                              n105 = Subtract(x=w696, y=sgl 90.0) -> (x-y=w694:sgl)
                            }
                            frame True {
                              # "Positive Y"
                              # "A2 is < 90"
                              n106 = Subtract(x=sgl 90.0, y=w698) -> (x-y=w699:sgl)
                            }
                          }
                          "dA2" <- w686
                          n107 = expression code="(x/180.0)*pi" "degrees to radians"(w686) -> (w684:sgl)
                          n108 = expression code="(x/180.0)*pi" "degrees to radians"(w686) -> (w685:sgl)
                          n109 = Cosine(x=w684) -> (cos(x)=w682:sgl)
                          n110 = Sine(x=w685) -> (sin(x)=w683:sgl)
                          n111 = Multiply(x=w676, y=w682) -> (x*y=w678:sgl)
                          n112 = Multiply(x=w676, y=w683) -> (x*y=w680:sgl)
                          n113 = case shown="True" w681 {
                            tunnel: w680 -> [w691 w692]
                            tunnel: [w690 w692] -> w677
                            frame False {
                              n114 = Negate(x=w691) -> (-x=w690:sgl)
                            }
                            frame True {
                            }
                          }
                        }
                      }
                    }
                    n115 = Boolean To (0,1)(Boolean=w305) -> (0, 1=w319:i16[])
                    n116 = Add Array Elements(numeric array=w319) -> (sum=w303:i16)
                    n117 = Greater?(x=w303, y=1) -> (0:w307:bool)
                    n118 = Bundle(w324, w323) -> (→"LOCAL\nBeacon Coordinates\nRelative to Robot" →"Local Coordinates - Calculated":cluster{sgl[], sgl[]})  [unwired: 1 in]
                    n119 = call "Coordinate_Outlier_Filtering_R2.vi"("Num of Beacons"=w298, "Max Std Dev(all 5)"="Max Std Dev (5)", "X in"=w324, "Valid Data\nSets in"=w309, "Y in"=w323, "Max Std Dev( 4 )"="Max Std Dev (4)", "Max Std Dev (3)"="Max Std Dev (3)") -> ("Y out"=w296:sgl[], "X out"=w297:sgl[], "Valid Beacons\nout"=w293:bool[], "Slope out"=w312:dbl)  [unwired: 3 in, 2 out]
                    n120 = Inverse Tangent(1:w312) -> (0:w336:dbl)
                    n121 = expression code="(x/pi)*180.0" "radians to degrees"(w336) -> (w311:dbl)
                    n122 = Boolean To (0,1)(Boolean=w293) -> (0, 1=w292:i16[])
                    n123 = To Single Precision Float(number=w311) -> (single precision float=w302:sgl)
                    "Orietnation\n(current)" <- w302
                    n124 = case shown="True" w307 {
                      tunnel: w305 -> [_ w402]
                      tunnel: [w378 w388] -> w304
                      tunnel: w306 -> [_ w389]
                      tunnel: w302 -> [w379 w383]
                      tunnel: [w377 w384] -> w301
                      tunnel: w294 -> [_ _]
                      frame False {
                        # "Since no history available,\ncheck that current is with 0-360"
                        # "Use Current Orientation bc \nPrevious are not available"
                        # "New Position\nValid"
                        n125 = In Range and Coerce(upper limit=sgl 360.0, x=w379, lower limit=sgl -360.0 ("upper limit")) -> (In Range?=w378:bool)  [unwired: 1 out]
                        n126 = Select(t=w379, s=w378, f=sgl 0.0) -> (s? t:f=w377:sgl)
                      }
                      frame True {
                        # "Valid Position Ccount\n(up to 2)"
                        # "Weighted\nOrientation"
                        # "New \nWeight"
                        # "Weighted Orientation (new)"
                        # "Position\nValid\n(current)\n\nbased on orientation"
                        # "Only Calculate MOving Avg\nif xx% of previous positions were valid"
                        n127 = Initialize Array(u8 0, u8 2) -> (w397:u8[])
                        n128 = local read "History Size"() -> (w398:u8)
                        n129 = while {
                          shift-right: [w453] -> w390
                          shift-left: w397 -> [w455]
                          tunnel: w402 -> [w462] mode=indexing
                          shift-right: [w460] -> w395
                          shift-left: u8 0 -> [w463]
                          tunnel: w398 -> [w461]
                          i -> [w454]
                          stop <- w456 stop-if-true
                          # "Grab Last 2 Valid Position Indexes"
                          n130 = case shown="True" w462 {
                            tunnel: w463 -> [w465 w467]
                            tunnel: [w465 w470] -> w460
                            tunnel: w455 -> [w464 w469]
                            tunnel: w454 -> [_ w468]
                            tunnel: [w464 w466] -> w453
                            frame False {
                            }
                            frame True {
                              # "Update Index\nto use"
                              # "Increment\nValid Count"
                              n131 = Replace Array Subset(array=w469, new element=w468, index=w467) -> (w466:u8[])
                              n132 = Increment(x=w467) -> (x+1=w470:u8)
                            }
                          }
                          n133 = Greater?(x=w454, y=w461) -> (0:w457:bool)
                          n134 = Greater?(x=w460, y=u8 2) -> (0:w458:bool)
                          n135 = Or(x=w458, y=w457) -> (x .or. y?=w456:bool)
                        }
                        n136 = case shown="2, Default" w395 {
                          tunnel: w390 -> [_ w437 w449]
                          tunnel: w389 -> [_ w438 w448]
                          tunnel: [sgl 0.0 ("y") w431 w444] -> w393
                          tunnel: "Orientation (-2) \nWeight" -> [w423 w434 w443]
                          tunnel: "Orientation (-1) \nWeight" -> [w425 w427 w441]
                          tunnel: "New Orientation\nWeight" -> [w424 w429 w442]
                          tunnel: [w422 w428 w442] -> w394
                          frame 0 {
                            n137 = Compound Arithmetic op=ADD(w425, w424, w423) -> (w422:sgl)
                          }
                          frame 1 {
                            # "Grab Last 1 Valid Position Values"
                            n138 = Index Array(array=w437, index=u8 0) -> (element=w435:u8)
                            n139 = Index Array(array=w438, index=w435) -> (element=w426:sgl)
                            n140 = Divide(x=w434, y=sgl 2.0) -> (x/y=w430:sgl)
                            n141 = Add(x=w427, y=w430) -> (x+y=w432:sgl)
                            n142 = Add(x=w430, y=w429) -> (x+y=w428:sgl)
                            n143 = Multiply(x=w426, y=w432) -> (x*y=w431:sgl)
                          }
                          frame 2, Default {
                            # "weighted vals"
                            # "Grab Last 2 Valid Position Values"
                            n144 = Index Array(array=w449, index=u8 0) -> (element=w451:u8)
                            n145 = Index Array(array=w449, index=u8 1) -> (element=w447:u8)
                            n146 = Index Array(array=w448, index=w451) -> (element=w440:sgl)
                            n147 = Index Array(array=w448, index=w447) -> (element=w439:sgl)
                            n148 = Multiply(x=w441, y=w440) -> (x*y=w445:sgl)
                            n149 = Multiply(x=w439, y=w443) -> (x*y=w446:sgl)
                            n150 = Add(x=w445, y=w446) -> (x+y=w444:sgl)
                          }
                        }
                        n151 = Multiply(x=w383, y=w394) -> (x*y=w392:sgl)
                        n152 = Add(x=w392, y=w393) -> (x+y=w391:sgl)
                        n153 = Greater Than 0?(x=w395) -> (x > 0?=w396:bool)
                        n154 = case shown="True" w396 {
                          tunnel: w391 -> [w405 w410]
                          tunnel: w390 -> [_ w418]
                          tunnel: w389 -> [_ w417]
                          tunnel: [w404 w409] -> w384
                          tunnel: [w403 w412] -> w388
                          frame False {
                            # "No Pevious is Available to Compare\ncheck that current is real angle"
                            n155 = In Range and Coerce(upper limit=sgl 360.0, x=w405, lower limit=sgl -360.0 ("upper limit")) -> (In Range?=w403:bool)  [unwired: 1 out]
                            n156 = Select(t=w405, s=w403, f=sgl 0.0) -> (s? t:f=w404:sgl)
                          }
                          frame True {
                            # "Calculate New, Weighted\nOrientation"
                            # "Check That New Value\nis within Range of Old\n(avg)"
                            # "(X1 - X2)^2"
                            # "Previous"
                            # "Pevious is Available to Compare"
                            n157 = Index Array(array=w418, index=u8 0) -> (element=w419:u8)
                            n158 = Index Array(array=w417, index=w419) -> (element=w415:sgl)
                            n159 = Subtract(x=w415, y=w410) -> (x-y=w414:sgl)
                            n160 = Absolute Value(x=w414) -> (abs(x)=w413:sgl)
                            n161 = Less Or Equal?(x=w413, y="New Orientation \nThreshold") -> (x <= y?=w412:bool)
                            n162 = Select(t=w410, s=w412, f=sgl 0.0) -> (s? t:f=w409:sgl)
                          }
                        }
                      }
                    }
                    n163 = Add Array Elements(numeric array=w292) -> (sum=w291:i16)
                    n164 = Greater?(x=w291, y=i16 2) -> (0:w289:bool)
                    n165 = case shown="True" w289 {
                      tunnel: w298 -> [_ w376]
                      tunnel: w293 -> [w369 w375]
                      tunnel: w297 -> [_ w374]
                      tunnel: w296 -> [_ w373]
                      tunnel: [w369 w372] -> w295
                      tunnel: "Distance\nBetween Beacons" -> [_ w371]
                      tunnel: "Distance\nBetween Beacons \n- Tolerance" -> [_ w370]
                      frame False {
                        # "Don't apply filtering,\nnot enough data points"
                      }
                      frame True {
                        # "This will filter beacons if they are calculate to be \ntoo close to each other. The beacon(s) that is\n discarded is chosen based distance between each/every\nbeacon,. Capable of filtering as long as 1/2 of sample\nset has uniform distances (between beacons)."
                        # "Validate Distance Between\nEach Beacon"
                        n166 = call "Beacon_Filtering_Inter_Beacon_Distance_R1.vi"("Num of Beacons"=w376, "Inter Beacon\nReal Distance"=w371, "X in"=w374, "Inter Beacon\ndelta Threshold"=w370, "Y in"=w373, "Valid Data\nSets in"=w375) -> ("Beacons Valid - Out"=w372:bool[])  [unwired: 9 in]
                      }
                    }
                    "Post Filtering\n- Valid Beacons" <- w295
                    n167 = Bundle("X out"=w297, "Y out"=w296) -> (→"Normalized Beacons\nCoordinates Relative\nto Robot\n- Local" →"Local Coordinates - Adjusted":cluster{"X out":sgl[], "Y out":sgl[]})  [unwired: 1 in]
                    n168 = Increment(x=w298) -> (x+1=w362:i8)
                    n169 = for {
                      N: w362 -> [_]
                      tunnel: [w658] -> w364 mode=indexing
                      tunnel: w297 -> [w654]
                      tunnel: w296 -> [w657]
                      tunnel: [w656] -> w365 mode=indexing
                      tunnel: w331 -> [w653]
                      i -> [w655]
                      # "Build Array's of Coordinates\nFor All Objects"
                      n170 = Greater Than 0?(x=w655) -> (x > 0?=w659:bool)
                      n171 = case shown="True" w659 {
                        tunnel: [w661 w667] -> w658
                        tunnel: w654 -> [w664 _]
                        tunnel: w657 -> [w663 _]
                        tunnel: [w660 0.0] -> w656
                        tunnel: w655 -> [w665 _]
                        tunnel: w653 -> [_ w667]
                        frame True {
                          # "Rest of Array is\nBeacon Coordinates"
                          n172 = Decrement(x=w665) -> (x-1=w662:i32)
                          n173 = Index Array(array=w664, index=w662) -> (element=w661:sgl)
                          n174 = Index Array(array=w663, index=w662) -> (element=w660:sgl)
                        }
                        frame False {
                          # "First object is the\nother Camera\n\nthis coordinate\nis simply:\nx = 0\ny = distance btween cams"
                        }
                      }
                    }
                    n175 = Bundle(w364, w365) -> (→"All Object Coordinates \n- Local" →"Local Coordinates - Normalized":cluster{sgl[], dbl[]})  [unwired: 1 in]
                    n176 = expression code="(x/180.0)*pi" "degrees to radians"(w301) -> (w308:sgl)
                    n177 = call-poly <vilib>:"2D Cartesian Coordinate Rotation.vi"("theta"=w308, "Y"=w365, "X"=w364) -> ("Y Out"=w339:dbl[], "X Out"=w340:dbl[])  [unwired: 6 in, 1 out]
                    n178 = Bundle("X Out"=w340, "Y Out"=w339) -> (→"All Object Coordinates \n- Local - Rotated" →"Local Coordinates - Rotated":cluster{"X Out":dbl[], "Y Out":dbl[]})  [unwired: 1 in]
                    n179 = Index Array(array=w339, index=w361) -> (element=w332:dbl)
                    n180 = Index Array(array=w340, index=w361) -> (element=w360:dbl)
                    n181 = for {
                      N: w298 -> [_]
                      tunnel: w339 -> [w649]
                      tunnel: w340 -> [w650]
                      tunnel: w360 -> [w648]
                      tunnel: w332 -> [w647]
                      tunnel: [w646] -> w328 mode=indexing
                      tunnel: [w645] -> w327 mode=indexing
                      tunnel: [w644] -> w286 mode=indexing
                      tunnel: [w643] -> w329 mode=indexing
                      i -> [w652]
                      n182 = Increment(x=w652) -> (x+1=w651:i32)
                      n183 = Index Array(array=w649, index=w651) -> (element=w643:dbl)
                      n184 = Index Array(array=w650, index=w651) -> (element=w644:dbl)
                      n185 = Subtract(x=w643, y=w647) -> (x-y=w645:dbl)
                      n186 = Subtract(x=w644, y=w648) -> (x-y=w646:dbl)
                    }
                    n187 = Bundle(w328, w327) -> (→"dX, dY\nRight Cam":cluster{dbl[], dbl[]})  [unwired: 1 in]
                    n188 = Bundle(w286, w329) -> (→"dX, dY\nLeft Cam":cluster{dbl[], dbl[]})  [unwired: 1 in]
                    n189 = Unbundle("Real Beacon\n - Coordinates") -> ("X"=w357:dbl[], "Y"=w333:dbl[])
                    n190 = Boolean To (0,1)(Boolean=w295) -> (0, 1=w330:i16[])
                    n191 = for {
                      N: w298 -> [_]
                      tunnel: w295 -> [w629] mode=indexing
                      tunnel: w357 -> [w626] mode=indexing
                      tunnel: w333 -> [w625] mode=indexing
                      tunnel: w286 -> [w628] mode=indexing
                      tunnel: w329 -> [w624] mode=indexing
                      tunnel: w328 -> [w627] mode=indexing
                      tunnel: w327 -> [w623] mode=indexing
                      tunnel: [w622] -> w356 mode=indexing
                      tunnel: [w621] -> w355 mode=indexing
                      tunnel: [w620] -> w354 mode=indexing
                      tunnel: [w619] -> w353 mode=indexing
                      n192 = case shown="True" w629 {
                        tunnel: w628 -> [_ w642]
                        tunnel: w627 -> [_ w641]
                        tunnel: w626 -> [_ w632]
                        tunnel: w625 -> [_ w631]
                        tunnel: w624 -> [_ w640]
                        tunnel: w623 -> [_ w633]
                        tunnel: [w630 w638] -> w622
                        tunnel: [w630 w637] -> w621
                        tunnel: [w630 w636] -> w620
                        tunnel: [w630 w635] -> w619
                        frame False {
                          w630 = sgl 0.0
                          # "Add Nothing"
                        }
                        frame True {
                          # "realX = beaconX + dY\nrealY = beaconY + (-dx)"
                          # "Right Cam"
                          # "Left Cam"
                          # "dX = -dX\nSwap dX, dY"
                          # "Translate to Real Coordinates\nOnly Apply for Valid Beacons"
                          n193 = Negate(x=w642) -> (-x=w639:dbl)
                          n194 = Negate(x=w641) -> (-x=w634:dbl)
                          n195 = Add(x=w632, y=w640) -> (x+y=w638:dbl)
                          n196 = Add(x=w631, y=w639) -> (x+y=w637:dbl)
                          n197 = Add(x=w632, y=w633) -> (x+y=w636:dbl)
                          n198 = Add(x=w631, y=w634) -> (x+y=w635:dbl)
                        }
                      }
                    }
                    n199 = Add Array Elements(numeric array=w330) -> (sum=w334:i16)
                    n200 = Add Array Elements(numeric array=w356) -> (sum=w352:dbl)
                    n201 = Add Array Elements(numeric array=w355) -> (sum=w351:dbl)
                    n202 = Add Array Elements(numeric array=w354) -> (sum=w350:dbl)
                    n203 = Add Array Elements(numeric array=w353) -> (sum=w349:dbl)
                    n204 = Divide(x=w352, y=w334) -> (x/y=w347:dbl)
                    n205 = Divide(x=w351, y=w334) -> (x/y=w345:dbl)
                    n206 = Divide(x=w350, y=w334) -> (x/y=w346:dbl)
                    n207 = Divide(x=w349, y=w334) -> (x/y=w344:dbl)
                    n208 = Bundle(w347, w345) -> (→"Left Camera Real Coordinates":cluster{dbl, dbl})  [unwired: 1 in]
                    n209 = Bundle(w346, w344) -> (→"Right Camera Real Coordinate":cluster{dbl, dbl})  [unwired: 1 in]
                    n210 = Add(x=w347, y=w346) -> (x+y=w343:dbl)
                    n211 = Add(x=w345, y=w344) -> (x+y=w341:dbl)
                    n212 = Divide(x=w343, y=w342) -> (x/y=w315:dbl)
                    n213 = Divide(x=w341, y=w342) -> (x/y=w314:dbl)
                    n214 = Bundle(w315, w314) -> (→"Robot Coordinates":cluster{dbl, dbl})  [unwired: 1 in]
                    n215 = case shown="True" w307 {
                      tunnel: w305 -> [_ w509]
                      tunnel: w303 -> [_ _]
                      tunnel: w315 -> [w475 w497]
                      tunnel: [w476 w487] -> w310
                      tunnel: w316 -> [_ w482]
                      tunnel: w314 -> [w474 w496]
                      tunnel: [w473 w508] -> w313
                      tunnel: "Max X (arena)" -> [w472 w485]
                      tunnel: "Max Y (arena)" -> [w471 w484]
                      frame False {
                        # "New Position\nValid"
                        # "Since no history available,\ncheck that current is within\nthe bounds of the arena size"
                        # "Use Current Position bc \nPrevious are not available"
                        n216 = In Range and Coerce(upper limit=w472, x=w475, lower limit=sgl 0.0 ("upper limit")) -> (In Range?=w478:bool)  [unwired: 1 out]
                        n217 = In Range and Coerce(upper limit=w471, x=w474, lower limit=sgl 0.0 ("upper limit")) -> (In Range?=w477:bool)  [unwired: 1 out]
                        n218 = Bundle(w475, w474) -> (w473:cluster{dbl, dbl})  [unwired: 1 in]
                        n219 = And(x=w478, y=w477) -> (x .and. y?=w476:bool)
                      }
                      frame True {
                        # "Only consider if velocity is\ngreater than certain speed"
                        # "Valid Position Ccount\n(up to 2)"
                        # "Weighted Y"
                        # "Weighted X"
                        # "New Pos\nWeight"
                        # "Weighted Robot \nCoordinates"
                        # "Position\nValid\n(current)"
                        # "Only Calculate MOving Avg\nif xx% of previous positions were valid"
                        n220 = Initialize Array(u8 0, u8 2) -> (w503:u8[])
                        n221 = local read "History Size"() -> (w504:u8)
                        n222 = while {
                          shift-right: [w602] -> w481
                          shift-left: w503 -> [w604]
                          tunnel: w509 -> [w610] mode=indexing
                          shift-right: [w608] -> w499
                          shift-left: u8 0 -> [w611]
                          tunnel: w504 -> [w609]
                          tunnel: [w601] -> w483
                          i -> [w603]
                          stop <- w605 stop-if-true
                          # "Grab Last 3 Valid Position Indexes"
                          n223 = case shown="True" w610 {
                            tunnel: w611 -> [w613 w615]
                            tunnel: [w613 w618] -> w608
                            tunnel: w604 -> [w612 w617]
                            tunnel: w603 -> [_ w616]
                            tunnel: [w612 w614] -> w602
                            frame False {
                            }
                            frame True {
                              # "Update Index\nto use"
                              # "Increment\nValid Count"
                              n224 = Replace Array Subset(array=w617, new element=w616, index=w615) -> (w614:u8[])
                              n225 = Increment(x=w615) -> (x+1=w618:u8)
                            }
                          }
                          n226 = Greater?(x=w603, y=w609) -> (0:w606:bool)
                          n227 = Greater?(x=w608, y=u8 2) -> (0:w601:bool)
                          n228 = Or(x=w601, y=w606) -> (x .or. y?=w605:bool)
                        }
                        n229 = case shown="True" w483 {
                          tunnel: w482 -> [_ w531]
                          tunnel: w481 -> [_ w517]
                          frame False {
                          }
                          frame True {
                            # "Angle between p(1) - p(2)"
                            # "Angle between p(0) - p(1)"
                            # "Calculate Orientation Based on Recent Positions"
                            # "*******"
                            n230 = Index Array(array=w517, index #1=0, index #2=1, index #3=2) -> (element #1=w513:u8, element #2=w512:u8, element #3=w511:u8)
                            n231 = Index Array(array=w531, index=w513) -> (element=w530:cluster{sgl, sgl})
                            n232 = Unbundle(w530) -> (w527:sgl, w526:sgl)
                            n233 = Index Array(array=w531, index=w512) -> (element=w529:cluster{sgl, sgl})
                            n234 = Unbundle(w529) -> (w519:sgl, w518:sgl)
                            n235 = Subtract(x=w527, y=w519) -> (x-y=w528:sgl)
                            n236 = Subtract(x=w526, y=w518) -> (x-y=w525:sgl)
                            n237 = Inverse Tangent (2 Input)(1:w525, 2:w528) -> (0:→"atan2(y,x)":sgl)
                            n238 = Index Array(array=w531, index=w511) -> (element=w520:cluster{sgl, sgl})
                            n239 = Unbundle(w520) -> (w523:sgl, w522:sgl)
                            n240 = Subtract(x=w519, y=w523) -> (x-y=w524:sgl)
                            n241 = Subtract(x=w518, y=w522) -> (x-y=w521:sgl)
                            n242 = Inverse Tangent (2 Input)(1:w521, 2:w524) -> ()  [unwired: 1 out]
                          }
                        }
                        n243 = case shown="2, Default" w499 {
                          tunnel: w481 -> [_ w578 w598]
                          tunnel: w482 -> [_ w579 w597]
                          tunnel: [w559 w568 w586] -> w495
                          tunnel: [w559 w567 w585] -> w494
                          tunnel: "position(-2) weight" -> [w561 w572 w584]
                          tunnel: "position(-1) weight" -> [w563 w570 w583]
                          tunnel: "New Position\nWeight" -> [w562 w565 w582]
                          tunnel: [w560 w564 w582] -> w498
                          frame 0 {
                            w559 = sgl 0.0 ("y")
                            n244 = Compound Arithmetic op=ADD(w563, w562, w561) -> (w560:sgl)
                          }
                          frame 1 {
                            # "Grab Last 1 Valid Position Values"
                            n245 = Index Array(array=w578, index=u8 0) -> (element=w576:u8)
                            n246 = Index Array(array=w579, index=w576) -> (element=w573:cluster{sgl, sgl})
                            n247 = Unbundle(w573) -> (w574:sgl, w575:sgl)
                            n248 = Divide(x=w572, y=sgl 2.0) -> (x/y=w566:sgl)
                            n249 = Add(x=w570, y=w566) -> (x+y=w569:sgl)
                            n250 = Add(x=w566, y=w565) -> (x+y=w564:sgl)
                            n251 = Multiply(x=w574, y=w569) -> (x*y=w568:sgl)
                            n252 = Multiply(x=w575, y=w569) -> (x*y=w567:sgl)
                          }
                          frame 2, Default {
                            # "weighted vals"
                            # "Grab Last 2 Valid Position Values"
                            n253 = Index Array(array=w598, index #1=u8 0, index #2=u8 1) -> (element #1=w599:u8, element #2=w580:u8)
                            n254 = Index Array(array=w597, index=w599) -> (element=w596:cluster{sgl, sgl})
                            n255 = Index Array(array=w597, index=w580) -> (element=w595:cluster{sgl, sgl})
                            n256 = Unbundle(w596) -> (w593:sgl, w594:sgl)
                            n257 = Unbundle(w595) -> (w592:sgl, w591:sgl)
                            n258 = Multiply(x=w593, y=w583) -> (x*y=w589:sgl)
                            n259 = Multiply(x=w594, y=w583) -> (x*y=w588:sgl)
                            n260 = Multiply(x=w592, y=w584) -> (x*y=w590:sgl)
                            n261 = Multiply(x=w591, y=w584) -> (x*y=w587:sgl)
                            n262 = Add(x=w589, y=w590) -> (x+y=w586:sgl)
                            n263 = Add(x=w588, y=w587) -> (x+y=w585:sgl)
                          }
                        }
                        n264 = Multiply(x=w497, y=w498) -> (x*y=w492:dbl)
                        n265 = Multiply(x=w496, y=w498) -> (x*y=w493:dbl)
                        n266 = Greater Than 0?(x=w499) -> (x > 0?=w500:bool)
                        n267 = Add(x=w492, y=w495) -> (x+y=w491:dbl)
                        n268 = Add(x=w493, y=w494) -> (x+y=w490:dbl)
                        n269 = case shown="True" w500 {
                          tunnel: w491 -> [w536 w543]
                          tunnel: w490 -> [w535 w542]
                          tunnel: w481 -> [_ w555]
                          tunnel: w482 -> [_ w554]
                          tunnel: [w533 w543] -> w489
                          tunnel: [w532 w542] -> w488
                          tunnel: [w537 w544] -> w487
                          tunnel: w485 -> [w539 _]
                          tunnel: w484 -> [w538 _]
                          frame False {
                            w534 = sgl 0.0 ("upper limit")
                            # "Check that within bounds of arena"
                            # "No Pevious is Available to Compare"
                            n270 = In Range and Coerce(upper limit=w539, x=w536, lower limit=w534) -> (In Range?=w541:bool)  [unwired: 1 out]
                            n271 = In Range and Coerce(upper limit=w538, x=w535, lower limit=w534) -> (In Range?=w540:bool)  [unwired: 1 out]
                            n272 = And(x=w541, y=w540) -> (x .and. y?=w537:bool)
                            n273 = Select(t=w536, s=w537, f=w534) -> (s? t:f=w533:dbl)
                            n274 = Select(t=w535, s=w537, f=w534) -> (s? t:f=w532:dbl)
                          }
                          frame True {
                            # "New"
                            # "(Y1 - Y2)^2"
                            # "(X1 - X2)^2"
                            # "Previous"
                            # "Pevious is Available to Compare"
                            n275 = Index Array(array=w555, index=u8 0) -> (element=w557:u8)
                            n276 = Index Array(array=w554, index=w557) -> (element=w556:cluster{sgl, sgl})
                            n277 = Unbundle(w556) -> (w546:sgl, w545:sgl)
                            n278 = Subtract(x=w546, y=w543) -> (x-y=w551:dbl)
                            n279 = Subtract(x=w542, y=w545) -> (x-y=w550:dbl)
                            n280 = Square(x=w551) -> (x^2=w549:dbl)
                            n281 = Square(x=w550) -> (x^2=w548:dbl)
                            n282 = Add(x=w549, y=w548) -> (x+y=w552:dbl)
                            n283 = Square Root(x=w552) -> (sqrt(x)=w547:dbl)
                            n284 = Less Or Equal?(x=w547, y="New Position \nThreshold") -> (x <= y?=w544:bool)
                          }
                        }
                        n285 = Bundle("upper limit"=w489, "upper limit"=w488) -> (w508:cluster{"upper limit":dbl, "upper limit":dbl})  [unwired: 1 in]
                      }
                    }
                    n286 = Less Than 0?(x=w314) -> ()  [unwired: 1 out]
                  }
                }
              }
            }
          }
        }
        n287 = And(x=w124, y=w123) -> (x .and. y?=w128:bool)
        "Position Valid" <- w128
        n288 = Exclusive Or(1:w123, 2:w124) -> (0:w122:bool)
        n289 = case shown="True" w128 {
          tunnel: [w163 w166] -> w142
          tunnel: [w164 w165] -> w127
          tunnel: w144 -> [_ w166]
          tunnel: w143 -> [_ w165]
          tunnel: w122 -> [_ _]
          frame False {
            w163 = sgl 0.0 ("f")
            n290 = Bundle("f"=w163, "f"=w163) -> (w164:cluster{"f":sgl, "f":sgl})  [unwired: 1 in]
          }
          frame True {
            # "For Servos"
            "Last Orientation" <- w166
            "Last Position" <- w165
          }
        }
        "Robot Coordinates - Avgd" <- w127
        "Orientation Avgd" <- w142
        n291 = local read "History Size"() -> (w134:u8)
        n292 = Reverse 1D Array(array=w141) -> (reversed array=w147:cluster{sgl, sgl}[])
        n293 = for {
          N: w134 -> [w204]
          shift-right: [w205] -> w148
          shift-left: w147 -> [w200]
          tunnel: w127 -> [w199]
          i -> [w201]
          n294 = Decrement(x=w204) -> (x-1=w202:i32)
          n295 = Equal?(x=w202, y=w201) -> (x = y?=w203:bool)
          n296 = case shown="True" w203 {
            tunnel: w201 -> [w207 w212]
            tunnel: w200 -> [w210 w213]
            tunnel: [w208 w214] -> w205
            tunnel: w199 -> [_ w211]
            frame False {
              n297 = Increment(x=w207) -> (x+1=w206:i32)
              n298 = Index Array(array=w210, index=w206) -> (element=w209:cluster{sgl, sgl})
              n299 = Replace Array Subset(array=w210, new element=w209, index=w207) -> (w208:cluster{sgl, sgl}[])
            }
            frame True {
              n300 = Replace Array Subset(array=w213, new element=w211, index=w212) -> (w214:cluster{sgl, sgl}[])
            }
          }
        }
        n301 = Reverse 1D Array(array=w140) -> (reversed array=w149:sgl[])
        n302 = Reverse 1D Array(array=w148) -> (reversed array=w137:cluster{sgl, sgl}[])
        n303 = for {
          N: w134 -> [w188]
          shift-right: [w189] -> w150
          shift-left: w149 -> [w184]
          tunnel: w142 -> [w183]
          i -> [w185]
          n304 = Decrement(x=w188) -> (x-1=w186:i32)
          n305 = Equal?(x=w186, y=w185) -> (x = y?=w187:bool)
          n306 = case shown="True" w187 {
            tunnel: w185 -> [w191 w196]
            tunnel: w184 -> [w194 w197]
            tunnel: [w192 w198] -> w189
            tunnel: w183 -> [_ w195]
            frame False {
              n307 = Increment(x=w191) -> (x+1=w190:i32)
              n308 = Index Array(array=w194, index=w190) -> (element=w193:sgl)
              n309 = Replace Array Subset(array=w194, new element=w193, index=w191) -> (w192:sgl[])
            }
            frame True {
              n310 = Replace Array Subset(array=w197, new element=w195, index=w196) -> (w198:sgl[])
            }
          }
        }
        n311 = Reverse 1D Array(array=w139) -> (reversed array=w145:bool[])
        n312 = Reverse 1D Array(array=w150) -> (reversed array=w138:sgl[])
        n313 = for {
          N: w134 -> [w172]
          shift-right: [w173] -> w146
          shift-left: w145 -> [w168]
          tunnel: w128 -> [w167]
          i -> [w169]
          n314 = Decrement(x=w172) -> (x-1=w170:i32)
          n315 = Equal?(x=w170, y=w169) -> (x = y?=w171:bool)
          n316 = case shown="True" w171 {
            tunnel: w169 -> [w175 w180]
            tunnel: w168 -> [w178 w181]
            tunnel: [w176 w182] -> w173
            tunnel: w167 -> [_ w179]
            frame False {
              n317 = Increment(x=w175) -> (x+1=w174:i32)
              n318 = Index Array(array=w178, index=w174) -> (element=w177:bool)
              n319 = Replace Array Subset(array=w178, new element=w177, index=w175) -> (w176:bool[])
            }
            frame True {
              n320 = Replace Array Subset(array=w181, new element=w179, index=w180) -> (w182:bool[])
            }
          }
        }
        n321 = Reverse 1D Array(array=w146) -> (reversed array=w133:bool[])
        n322 = Boolean To (0,1)(Boolean=w133) -> (0, 1=w132:i16[])
        n323 = Add Array Elements(numeric array=w132) -> (sum=w130:i16)
        n324 = Greater Or Equal?(x=w130, y=i16 2) -> (x >= y?=→"Position \nLock Status":bool)
        n325 = case shown="True" w128 {
          tunnel: w127 -> [_ w162]
          frame False {
          }
          frame True {
            # "update debug graph\nif current is valid"
            n326 = Unbundle(w162) -> ("upper limit"=w161:dbl, "upper limit"=w160:dbl)
            n327 = Build Array(w160) -> (w158:dbl[])
            n328 = Build Array(w161) -> (w159:dbl[])
            n329 = Bundle(w159, w158) -> (→"Real Position in Course 2":cluster{dbl[], dbl[]})  [unwired: 1 in]
          }
        }
      }
    }
    n330 = case shown="True" w97 {
      tunnel: w96 -> [_ w104]
      frame False {
      }
      frame True {
        n331 = call "Tick Count3"() -> ("Tick Count(uSec)"=w105:u32)
        n332 = Subtract(x=w105, y=w104) -> (x-y=w108:u32)
        n333 = Divide(x=w108, y=u32 1000 ("x")) -> (x/y=→"dT":dbl)
      }
    }
    n334 = call "Tick Count6"() -> ("Tick Count(uSec)"=w94:u32)
    "Robot Coordinates\nHistory" <- w93
    "Orientation\nHistory" <- w98
    "Position Valid\nHistory" <- w99
  }
  n335 = disable-structure shown="Disabled" {
    frame Disabled {
      w733 = sgl 0.0
      # "Y"
      # "X"
      n336 = Bundle(w733, w733) -> (w730:cluster{sgl, sgl})  [unwired: 1 in]
      n337 = Initialize Array(w733, 10 ("dimension size")) -> (w727:sgl[])
      n338 = Initialize Array(FALSE, 10 ("dimension size")) -> (w728:bool[])
      n339 = local read "Real Beacon\n - Coordinates"() -> (w734:cluster{"X":dbl[], "Y":dbl[]})
      n340 = Unbundle(w734) -> ("X"=w732:dbl[], "Y"=w731:dbl[])
      n341 = while {
        shift-right: [w760] -> _
        shift-left: w727 -> [w761]
        shift-right: [w744] -> _
        shift-left: w728 -> [w764]
        shift-right: [w746] -> _
        shift-left: w727 -> [w765]
        shift-right: [w747] -> _
        shift-left: w730 -> [w749]
        shift-right: [w743] -> _
        shift-left: FALSE -> [w748]
        tunnel: w732 -> [w740]
        tunnel: w731 -> [w739]
        stop <- FALSE stop-if-true
        w745 = 0
        w757 = 5
        # "Update Shift Regs"
        # "Update Shift Arrays"
        n342 = local read "Robot Coordinates"() -> (w753:cluster{"X":sgl, "Y":sgl})
        n343 = local read "Position Valid"() -> (w754:bool)
        n344 = Unbundle(w753) -> ("X"=w763:sgl, "Y"=w762:sgl)
        n345 = Reverse 1D Array(array=w764) -> (reversed array=w766:bool[])
        n346 = Reverse 1D Array(array=w765) -> (reversed array=w772:sgl[])
        n347 = Reverse 1D Array(array=w761) -> (reversed array=w769:sgl[])
        n348 = for {
          N: 10 -> [w861]
          shift-right: [w862] -> w774
          shift-left: w772 -> [w857]
          tunnel: w763 -> [w856]
          i -> [w858]
          n349 = Decrement(x=w861) -> (x-1=w859:i32)
          n350 = Equal?(x=w859, y=w858) -> (x = y?=w860:bool)
          n351 = case shown="True" w860 {
            tunnel: w858 -> [w864 w869]
            tunnel: w857 -> [w867 w870]
            tunnel: [w865 w871] -> w862
            tunnel: w856 -> [_ w868]
            frame False {
              n352 = Increment(x=w864) -> (x+1=w863:i32)
              n353 = Index Array(array=w867, index=w863) -> (element=w866:sgl)
              n354 = Replace Array Subset(array=w867, new element=w866, index=w864) -> (w865:sgl[])
            }
            frame True {
              n355 = Replace Array Subset(array=w870, new element=w868, index=w869) -> (w871:sgl[])
            }
          }
        }
        n356 = for {
          N: 10 -> [w845]
          shift-right: [w846] -> w771
          shift-left: w769 -> [w841]
          tunnel: w762 -> [w840]
          i -> [w842]
          n357 = Decrement(x=w845) -> (x-1=w843:i32)
          n358 = Equal?(x=w843, y=w842) -> (x = y?=w844:bool)
          n359 = case shown="True" w844 {
            tunnel: w842 -> [w848 w853]
            tunnel: w841 -> [w851 w854]
            tunnel: [w849 w855] -> w846
            tunnel: w840 -> [_ w852]
            frame False {
              n360 = Increment(x=w848) -> (x+1=w847:i32)
              n361 = Index Array(array=w851, index=w847) -> (element=w850:sgl)
              n362 = Replace Array Subset(array=w851, new element=w850, index=w848) -> (w849:sgl[])
            }
            frame True {
              n363 = Replace Array Subset(array=w854, new element=w852, index=w853) -> (w855:sgl[])
            }
          }
        }
        n364 = for {
          N: 10 -> [w829]
          shift-right: [w830] -> w768
          shift-left: w766 -> [w825]
          tunnel: w754 -> [w824]
          i -> [w826]
          n365 = Decrement(x=w829) -> (x-1=w827:i32)
          n366 = Equal?(x=w827, y=w826) -> (x = y?=w828:bool)
          n367 = case shown="False" w828 {
            tunnel: w826 -> [w832 w837]
            tunnel: w825 -> [w835 w838]
            tunnel: [w833 w839] -> w830
            tunnel: w824 -> [_ w836]
            frame False {
              n368 = Increment(x=w832) -> (x+1=w831:i32)
              n369 = Index Array(array=w835, index=w831) -> (element=w834:bool)
              n370 = Replace Array Subset(array=w835, new element=w834, index=w832) -> (w833:bool[])
            }
            frame True {
              n371 = Replace Array Subset(array=w838, new element=w836, index=w837) -> (w839:bool[])
            }
          }
        }
        n372 = Reverse 1D Array(array=w768) -> (reversed array=w744:bool[])
        n373 = Reverse 1D Array(array=w771) -> (reversed array=w760:sgl[])
        n374 = Reverse 1D Array(array=w774) -> (reversed array=w746:sgl[])
        n375 = Boolean To (0,1)(Boolean=w744) -> (0, 1=w759:i16[])
        n376 = Add Array Elements(numeric array=w759) -> (sum=w752:i16)
        n377 = Greater Or Equal?(x=w752, y=3) -> (x >= y?=w750:bool)
        n378 = case shown="True" w750 {
          tunnel: w760 -> [_ w793]
          tunnel: w746 -> [_ w792]
          tunnel: w744 -> [_ w787]
          tunnel: w752 -> [_ w786]
          tunnel: [w778 w779] -> w747
          tunnel: w749 -> [w778 w785]
          tunnel: "New Pos\nThreshold (*unit)\nfilterd UNUSED" -> [_ w784]
          tunnel: w748 -> [_ w783]
          tunnel: [FALSE w782] -> w743
          tunnel: [w776 w781] -> w742
          tunnel: [w776 w780] -> w741
          frame False {
            w776 = sgl 0.0
            # "false bc did not meet\ncriteria for enough previous \nvalid positions"
            # "Retain Last Valid Position Value"
          }
          frame True {
            w791 = sgl 0.0
            # "Only Calculate MOving Avg\nif xx% of previous positions were valid"
            n379 = for {
              N: 10 -> [_]
              tunnel: w787 -> [w815] mode=indexing
              tunnel: w793 -> [w814] mode=indexing
              tunnel: w792 -> [w813] mode=indexing
              shift-right: [w811] -> w789
              shift-left: w791 -> [w812]
              shift-right: [w809] -> w788
              shift-left: w791 -> [w810]
              # "Calculate Moving Average"
              n380 = case shown="True" w815 {
                tunnel: w814 -> [_ w819]
                tunnel: w813 -> [_ w822]
                tunnel: w812 -> [w817 w823]
                tunnel: [w817 w821] -> w811
                tunnel: w810 -> [w816 w820]
                tunnel: [w816 w818] -> w809
                frame False {
                }
                frame True {
                  n381 = Add(x=w823, y=w822) -> (x+y=w821:sgl)
                  n382 = Add(x=w820, y=w819) -> (x+y=w818:sgl)
                }
              }
            }
            n383 = Divide(x=w789, y=w786) -> (x/y=w781:sgl)
            n384 = Divide(x=w788, y=w786) -> (x/y=w780:sgl)
            n385 = Bundle(w781, w780) -> (w779:cluster{sgl, sgl})  [unwired: 1 in]
            n386 = case shown="True" w783 {
              tunnel: w785 -> [_ w798]
              tunnel: w779 -> [_ w797]
              tunnel: w784 -> [_ w796]
              tunnel: [TRUE w795] -> w782
              frame False {
                # "True bc this position has\nno previous position\nto compare to"
              }
              frame True {
                # "Previous Position"
                # "New (filtered) Position"
                # "Only Check If Close to previous position\nif previous position was valid"
                # "(Y1 - Y2)^2"
                # "(X1 - X2)^2"
                n387 = Unbundle(w798) -> (w806:sgl, w808:sgl)
                n388 = Unbundle(w797) -> (w805:sgl, w807:sgl)
                n389 = Subtract(x=w805, y=w806) -> (x-y=w803:sgl)
                n390 = Subtract(x=w807, y=w808) -> (x-y=w802:sgl)
                n391 = Square(x=w803) -> (x^2=w801:sgl)
                n392 = Square(x=w802) -> (x^2=w800:sgl)
                n393 = Add(x=w801, y=w800) -> (x+y=w804:sgl)
                n394 = Square Root(x=w804) -> (sqrt(x)=w799:sgl)
                n395 = Less?(x=w799, y=w796) -> (x < y?=w795:bool)
              }
            }
          }
        }
        n396 = Replace Array Subset(array=w746, new element=w742, index=w745) -> ()  [unwired: 1 out]
        n397 = Replace Array Subset(array=w744, new element=w743, index=w745) -> ()  [unwired: 1 out]
        n398 = Replace Array Subset(array=w746, new element=w741, index=w745) -> ()  [unwired: 1 out]
        n399 = Replace Array Subset(array=w740, new element=w742, index=w757) -> (w756:dbl[])
        n400 = Replace Array Subset(array=w739, new element=w741, index=w757) -> (w755:dbl[])
        n401 = call "Wait7"("Count(mSec)"=u32 200) -> ()  [unwired: 1 out]
      }
    }
    frame Enabled {
    }
  }
  n402 = Initialize Array(0, 5) -> (→"Array 2":i32[])
  n403 = To Word Integer(number=w15) -> (16bit integer=w17:i16)
  n404 = To Word Integer(number=w15) -> (16bit integer=w18:i16)
  n405 = call "Tick Count8"() -> ("Tick Count(uSec)"=w12:u32)
  n406 = while {
    shift-right: [w921] -> _
    shift-left: i8 3 -> [w923]
    shift-right: [w919] -> _
    shift-left: i8 0 -> [w920]
    tunnel: [w892] -> _
    tunnel: [w893] -> _
    shift-right: [w916] -> _
    shift-left: w16 -> [w917]
    shift-right: [w915] -> _
    shift-left: w15 -> [w880]
    shift-right: [w913] -> _
    shift-left: w16 -> [w914]
    shift-right: [w912] -> _
    shift-left: w15 -> [w876]
    shift-right: [w908] -> _
    shift-left: w18 -> [w910]
    shift-right: [w907] -> _
    shift-left: w17 -> [w909]
    shift-right: [w905] -> _
    shift-left: w1 -> [w904]
    shift-right: [w906] -> _
    shift-left: w1 -> [w903]
    shift-right: [w902] -> _
    shift-left: _ -> [_]
    shift-right: [w901] -> _
    shift-left: _ -> [_]
    shift-right: [w898] -> _
    shift-left: w15 -> [w899]
    shift-right: [w888] -> _
    shift-left: w15 -> [w900]
    shift-right: [w882] -> _
    shift-left: w12 -> [w883]
    shift-right: [w872] -> _
    shift-left: w1 -> [w875]
    stop <- FALSE stop-if-true
    # "Avoid Direction\nLatch"
    n407 = disable-structure shown="Enabled" {
      disable-tunnel: [w929 _] -> w892
      disable-tunnel: ["Search Step Size\n(deg)" _] -> w893
      frame Enabled {
        n408 = Multiply(x=3.413333333333333, y="Search Step Size\n(deg)") -> (x*y=w927:dbl)
        n409 = To Unsigned Word Integer(number=w927) -> (unsigned 16bit integer=w929:u16)
      }
      frame Disabled {
      }
    }
    n410 = call "Tick Count7"() -> ("Tick Count(uSec)"=w882:u32)
    n411 = Subtract(x=w882, y=w883) -> (x-y=w885:u32)
    n412 = Divide(x=w885, y=u32 1000) -> (x/y=→"dT - Logic Loop":dbl)
    n413 = Multiply(x="Move Servo\nThreshold (deg)", y=3.413333333333333) -> (x*y=w896:dbl)
    n414 = To Unsigned Word Integer(number=w896) -> (unsigned 16bit integer=w894:u16)
    n415 = local read "SERVO ENABLE"() -> (w918:bool)
    n416 = Greater Or Equal?(x=w880, y="Max Dual\nBad Count") -> (x >= y?=w879:bool)
    n417 = Greater Or Equal?(x=w876, y="Max Dual\nBad Count") -> (x >= y?=w878:bool)
    n418 = And(x=w879, y=w878) -> (x .and. y?=w874:bool)
    n419 = case shown="True" w875 {
      tunnel: w874 -> [w924 w926]
      tunnel: [w924 w925] -> w873
      frame False {
      }
      frame True {
        n420 = Not(x=w926) -> (.not. x?=w925:bool)
      }
    }
    n421 = case shown="True" w918 {
      tunnel: w923 -> [w940 w1053]
      tunnel: [w940 w1057] -> w921
      tunnel: w920 -> [w939 w1015]
      tunnel: [w939 w984] -> w919
      tunnel: w894 -> [_ w975]
      tunnel: "Wait Count\nFactor" -> [_ w1013]
      tunnel: w892 -> [_ w1010]
      tunnel: w893 -> [_ _]
      tunnel: w917 -> [w938 w1035]
      tunnel: w880 -> [_ w1052]
      tunnel: [w938 w1034] -> w916
      tunnel: [w932 w1051] -> w915
      tunnel: "Start Search\nThreshold\n (x Wait Thres)" -> [_ w1012]
      tunnel: w876 -> [_ w1016]
      tunnel: w914 -> [w936 w991]
      tunnel: [w936 w988] -> w913
      tunnel: [w932 w985] -> w912
      tunnel: w910 -> [_ w1039]
      tunnel: w909 -> [_ w983]
      tunnel: [w933 w978] -> w908
      tunnel: [w933 w979] -> w907
      tunnel: [w931 w1041] -> w906
      tunnel: [w931 w980] -> w905
      tunnel: w904 -> [_ w1011]
      tunnel: w903 -> [_ w1040]
      tunnel: "Max delta Angle" -> [_ w974]
      tunnel: w900 -> [_ w1008]
      tunnel: w899 -> [_ w1017]
      tunnel: [w933 w1019] -> w898
      tunnel: [w933 w1007] -> w888
      tunnel: "Max Smart \nSearch Attempts" -> [_ w972]
      tunnel: "Max Search\n- Reactive Search Timeout" -> [_ w971]
      tunnel: w873 -> [_ w964]
      tunnel: w875 -> [_ w965]
      tunnel: [w931 w964] -> w872
      frame False {
        (unwired) 0
        w931 = FALSE
        w933 = 0
        # "Servo Disabled"
        # "Reset All Counters"
        n422 = case shown="True" "MANUAL SERVO \nCONTROL ENABLE" {
          frame False {
          }
          frame True {
            # "45 DEG MOUNT OFFSET"
            # "45 DEG MOUNT OFFSET"
            n423 = Add(x="Right Manual\nAngle", y=sgl 45.0) -> (x+y=w946:sgl)
            n424 = Subtract(x="Left Manual\nAngle", y=sgl 45.0) -> (x-y=w954:sgl)
            n425 = Add(x=w946, y=sgl 60.0) -> (x+y=w948:sgl)
            n426 = Add(x=w954, y=sgl 60.0) -> (x+y=w956:sgl)
            n427 = Multiply(x=3.413333333333333, y=w948) -> (x*y=w950:dbl)
            n428 = Multiply(x=3.413333333333333, y=w956) -> (x*y=w958:dbl)
            n429 = Add(x=0.5, y=w950) -> (x+y=w952:dbl)
            n430 = Add(x=0.5, y=w958) -> (x+y=w960:dbl)
            n431 = To Unsigned Word Integer(number=w952) -> (unsigned 16bit integer=w943:u16)
            n432 = To Unsigned Word Integer(number=w960) -> (unsigned 16bit integer=w942:u16)
            n433 = local write "Servo Goal Position\n - Left"(w942) -> ()
            n434 = local write "Servo Goal Position\n - Right"(w943) -> ()
          }
        }
        n435 = local read "Max Smart \nSearch Attempts"() -> (w935:i32)
        n436 = Subtract(x=w935, y=3) -> (x-y=w932:i32)
      }
      frame True {
        w998 = u16 1023
        w1043 = u16 1023
        # "Current Direction"
        # "Complete Search Mode\nMove Servos in Opposite Direction"
        # "Complete Search Mode\nMove Servos in Opposite Direction"
        # "Left Servo Track \nAngle Valid?"
        # "Start \nSearch\nThreshold"
        # "Reactive Search\nTimeout"
        # "Reactive Search\nTimeout"
        # "Manually Reset\nRespond Flag"
        # "Over-ride Direction"
        # "Manuallly Reset\nRespond Var"
        # "Manuallly Reset\nRespond Var"
        # "Direction Override"
        # "Move Servo and Tracking"
        # "*Note* Directions (for this case)\nare opposite for each servo!"
        # "Update Last Known Track Position \n& Update delta (move) position"
        # "Update Known Track Angle"
        # "Max Threhsold"
        # "Current Direction"
        # "Wait Count"
        # "Search Cycle Count"
        # "delta (move) angle, specific to last trackin angle"
        # "Current Goal Posiiton \nminus Last Known Track\nAngle"
        # "If Current Angle Valid\n& Move Servo = T\n& Out of Range of Last Track Angle\n& Other Servo Not Moving\n\nThen Update delta Move Angle"
        # "Move Servo? -R"
        # "Move Threhsold"
        # "Current Position"
        # "Last Known Track Angle"
        # "Apply Ceiling"
        # "Current Servo Goal Position"
        # "Only Move Servo if\nGoal Position  is out of range\nof Current Position and\nlast known track angle and\nnot too big of a change"
        # "If Already Parallel to Other Side,\nMove Servo *5* deg"
        # "Pan if Already at Parallel Angle\nor if Past deltaPan"
        # "Update Comm Process Variables"
        # "Both Tracking"
        # "Current delta - L"
        # "delta move sum - R"
        # "delta move sum - L"
        # "Current delta - R"
        # "Service Move Respond Variables"
        # "Direction Override"
        # "Move Servo and Tracking"
        # "Manually Reset\nRespond Flag"
        # "*Note* Directions (for this case)\nare opposite for each servo!"
        # "Over-ride Direction"
        # "Update Last Known Track Position \n& Update delta (move) position"
        # "Update Known Track Angle"
        # "delta Move Angle - R\n(Sum)"
        # "Search Step\nSize"
        # "Move Respond"
        # "Move Respond"
        # "Wait Cycle Threshold"
        # "Max Threhsold"
        # "Search Cycle Count - R"
        # "delta Move Angle -L\n(Sum)"
        # "Search Step\nSize"
        # "Wait Count"
        # "Search Cycle Count"
        # "DATA BUS AREA"
        # "delta (move) angle, specific to last trackin angle"
        # "Current Goal Posiiton \nminus Last Known Track\nAngle"
        # "If Current Angle Valid\n& Move Servo = T\n& Out of Range of Last Track Angle\n& Other Servo Not Moving\n\nThen Update delta Move Angle"
        # "Move Servo? -L"
        # "Move Threhsold"
        # "Current Position"
        # "Last Known Track Angle"
        # "Apply Ceiling"
        # "Current Servo Goal Position"
        # "\"Track\" if tracking angle is available,\nor\nwait until timeout & Search"
        # "Only Move Servo if\nGoal Position  is out of range\nof Current Position and\nlast known track angle and\nnot too big of a change"
        # "Tracking Angle\nAvailable?"
        n437 = local read "Current R (10bit)"() -> (w976:u16)
        n438 = Not(x=w965) -> (.not. x?=w970:bool)
        n439 = local read "Current L (10bit)"() -> (w1056:u16)
        n440 = case shown="False" "Angles Valid - R" {
          tunnel: w1015 -> [w1093 _]
          tunnel: [w1095 w1292] -> w992
          tunnel: [w1094 i8 0] -> w984
          tunnel: w1013 -> [w1078 _]
          tunnel: w976 -> [w1092 _]
          tunnel: [w1091 u16 0] -> w985
          tunnel: w1016 -> [w1090 _]
          tunnel: w1012 -> [w1088 _]
          tunnel: w1010 -> [w1087 _]
          tunnel: w1011 -> [w1086 _]
          tunnel: w983 -> [w1085 _]
          tunnel: [FALSE TRUE] -> w986
          tunnel: "Angles Valid - L" -> [w1083 _]
          tunnel: [w1082 FALSE] -> w977
          tunnel: [w1081 FALSE] -> w973
          tunnel: w1008 -> [w1080 _]
          tunnel: [w1079 0] -> w1007
          tunnel: w972 -> [w1077 _]
          tunnel: w971 -> [w1076 _]
          tunnel: w970 -> [w1075 _]
          frame False {
            # "Wait Cycle Threshold"
            # "Wait Threshold Multiplier"
            # "Wait # of 'ticks' until\n1 wait cycle\n\n1 Wait Cycle is equal to\n= Servo Algorithm Cycle Time X Wait Time Factor"
            # "Searching Logic"
            n441 = Greater Or Equal?(x=w1093, y=w1078) -> (x >= y?=w1089:bool)
            n442 = case shown="True" w1089 {
              tunnel: [w1102 w1122] -> w1095
              tunnel: [w1099 i8 0] -> w1094
              tunnel: w1093 -> [w1101 _]
              tunnel: w1092 -> [w1102 w1121]
              tunnel: [w1100 w1115] -> w1091
              tunnel: w1090 -> [w1100 w1114]
              tunnel: w1088 -> [_ w1113]
              tunnel: w1087 -> [_ w1119]
              tunnel: w1086 -> [_ w1107]
              tunnel: w1085 -> [_ w1118]
              tunnel: w1083 -> [_ w1117]
              tunnel: [FALSE w1116] -> w1082
              tunnel: [FALSE w1111] -> w1081
              tunnel: w1080 -> [w1096 w1110]
              tunnel: [w1096 w1109] -> w1079
              tunnel: w1077 -> [_ w1105]
              tunnel: w1076 -> [_ w1104]
              tunnel: w1075 -> [_ w1103]
              frame False {
                # "F"
                # "Current Servo Position (UINT 10)"
                # "Search Cycle Count (Don't update)"
                # "Wait Cycle Count"
                # "Increment Wait Cycle Counter, \nwait until counter is finished"
                n443 = Increment(x=w1101) -> (x+1=w1099:i8)
              }
              frame True {
                # "Reset Wait\nCount"
                # "Wait Until Start\nSearch Threshold\nto Begin Smart Search"
                # "Increment Search\n Cycle Count"
                # "Start Search Threshold..\n\nCould be added to further delay\nregular search"
                n444 = Greater Or Equal?(x=w1114, y=w1113) -> (x >= y?=w1106:bool)
                n445 = Or(x=w1106, y=w1107) -> (x .or. y?=w1108:bool)
                n446 = case shown="True" w1108 {
                  tunnel: [w1126 w1143] -> w1122
                  tunnel: w1121 -> [w1126 w1142]
                  tunnel: [w1125 w1141] -> w1120
                  tunnel: w1119 -> [_ w1140]
                  tunnel: w1118 -> [_ w1139]
                  tunnel: w1107 -> [_ w1138]
                  tunnel: w1117 -> [_ w1133]
                  tunnel: [FALSE w1137] -> w1116
                  tunnel: w1114 -> [w1125 w1136]
                  tunnel: [FALSE w1135] -> w1111
                  tunnel: w1110 -> [w1123 w1132]
                  tunnel: [w1123 w1131] -> w1109
                  tunnel: w1105 -> [_ w1130]
                  tunnel: w1104 -> [_ w1129]
                  tunnel: w1103 -> [_ _]
                  frame False {
                    # "F"
                    # "Do Nothing, \nwait until Search Count is Above Threshold"
                  }
                  frame True {
                    # "Add feature to \nonly attempt smart seach\ncertain number of times instead\nof waiting until certain number\nof searches to switch to\nthe generic search"
                    # "Or if Other Servo\nHas Trackin Info"
                    # "Only Attempt\nSmart Search \nUntil This count"
                    # "Current Servo Position"
                    n447 = Less?(x=w1136, y=w1130) -> (x < y?=w1134:bool)
                    n448 = Compound Arithmetic op=OR(w1134, w1133) -> (w1128:bool)
                    n449 = case shown="True" w1128 {
                      tunnel: [w1156 w1255] -> w1143
                      tunnel: w1142 -> [w1152 w1258]
                      tunnel: [w1153 w1249] -> w1141
                      tunnel: w1140 -> [w1148 w1251]
                      tunnel: w1138 -> [w1147 _]
                      tunnel: w1139 -> [w1157 _]
                      tunnel: w1136 -> [w1153 w1249]
                      tunnel: w1133 -> [w1155 _]
                      tunnel: [w1154 FALSE] -> w1137
                      tunnel: [w1151 FALSE] -> w1135
                      tunnel: w1132 -> [w1150 w1247]
                      tunnel: [w1149 w1247] -> w1131
                      tunnel: w1129 -> [w1146 _]
                      frame True {
                        # "SMART SEARCH"
                        # "********************\nUser seperate count for\nthis case to ensure\nthat this is attempted\nat least *3* times before\ntrying Recovery Search"
                        # "******************************\ninstead of limiting when reactive\ncan occur... maybe just have this number\nset the preference for which\nrecovery technique to use"
                        # "Search Must Be\nLess than this to Attempt\nReactive Recovery Search\n\nWill Attempt Recovery Search\nAfter This"
                        # "Search Goal\nPosition"
                        # "Move Respond - L"
                        # "Check if other\nservo moved\n& Search"
                        # "Since first time searching \nsince previously tracking,\n if this servo hasn't responded to other's last movement\nUse it to Predict where to begin Search"
                        n450 = Less?(x=w1153, y=w1146) -> (x < y?=w1145:bool)
                        n451 = And(x=w1147, y=w1145) -> (x .and. y?=w1144:bool)
                        n452 = case shown="False" w1144 {
                          tunnel: w1152 -> [_ w1206]
                          tunnel: w1157 -> [_ w1207]
                          tunnel: [w1164 w1201] -> w1156
                          tunnel: w1155 -> [w1159 _]
                          tunnel: [w1165 FALSE] -> w1154
                          tunnel: w1152 -> [w1163 _]
                          tunnel: [FALSE TRUE] -> w1151
                          tunnel: w1150 -> [w1161 w1202]
                          tunnel: [w1160 w1202] -> w1149
                          tunnel: w1148 -> [w1158 _]
                          frame False {
                            # "Left Right Servo"
                            # "Left Servo Track \nAngle Valid?"
                            # "F"
                            # "Reactive Search Using Other Servo Feedback Not Available...\nAttempt Recovery Search if Other Servo is Tracking"
                            n453 = case shown="True" w1159 {
                              tunnel: [FALSE TRUE] -> w1165
                              tunnel: [w1166 w1170] -> w1164
                              tunnel: w1163 -> [w1166 w1175]
                              tunnel: w1161 -> [w1167 w1173]
                              tunnel: [w1167 w1172] -> w1160
                              tunnel: w1158 -> [_ w1169]
                              frame False {
                                # "No Info Available.... do nothin for now... maybe move a little"
                                # "F"
                              }
                              frame True {
                                # "Recover Search\nCount"
                                # "****************\n*************"
                                # "If 0, Set GP to parallel\n-increment count\nIf >0, Pan CW by step size/2\nIf > 5, reset count\n\nreset count in Track case too"
                                # "Check # of Times\nThis Case Has Been\nEntered"
                                n454 = Greater Than 0?(x=w1173) -> (x > 0?=w1174:bool)
                                n455 = case shown="True" w1174 {
                                tunnel: [w1178 w1192] -> w1170
                                tunnel: w1175 -> [_ w1193]
                                tunnel: w1173 -> [w1176 w1194]
                                tunnel: [w1177 w1195] -> w1172
                                tunnel: w1169 -> [_ w1190]
                                frame False {
                                # "Move Servo Parallel to Other Servo"
                                # "First Attempt at Recovery Search"
                                # "45 DEG MOUNT OFFSET"
                                # "1024/300"
                                n456 = local read "Middle Beacon\nAngle - Left"() -> (w1180:sgl)
                                n457 = Increment(x=w1176) -> (x+1=w1177:i32)
                                n458 = Add(x=w1180, y=sgl 45.0) -> (x+y=w1182:sgl)
                                n459 = Add(x=w1182, y=sgl 60.0) -> (x+y=w1184:sgl)
                                n460 = Multiply(x=3.413333333333333, y=w1184) -> (x*y=w1186:dbl)
                                n461 = Add(x=0.5, y=w1186) -> (x+y=w1179:dbl)
                                n462 = To Unsigned Word Integer(number=w1179) -> (unsigned 16bit integer=w1178:u16)
                                }
                                frame True {
                                # "sTEP siZE\nfine factor"
                                # "Attempt to Pan in Steps Towards other Servo"
                                # "Could be same or function of \nregular search step size"
                                # "CCW= add"
                                # "MAKE SURE ADDING/SUBTRACTING\nTO RIGHT DIRECTION"
                                # "Search Count Greater Than 0"
                                n463 = Greater Or Equal?(x=w1194, y=u16 10) -> (x >= y?=w1196:bool)
                                n464 = case shown="False" w1196 {
                                tunnel: [w1198 u16 0 ("y")] -> w1195
                                tunnel: w1194 -> [w1199 _]
                                frame False {
                                # "Increment Count"
                                # "Continue to Pan until Limit Reached"
                                n465 = Increment(x=w1199) -> (x+1=w1198:i32)
                                }
                                frame True {
                                # "Count (pan attempts) limit reached\n\nReset Count"
                                }
                                }
                                n466 = Divide(x=w1190, y=u16 3) -> (x/y=w1189:dbl)
                                n467 = To Unsigned Word Integer(number=w1189) -> (unsigned 16bit integer=w1188:u16)
                                n468 = Add(x=w1193, y=w1188) -> (x+y=w1192:u16)
                                }
                                }
                              }
                            }
                          }
                          frame True {
                            # "Reactive Recovery Search using Other Servo Elapsed Movements"
                            # "Other Servo Has Moved - Use History of Other Servo to Estimate Search Start Position"
                            # "** check this"
                            # "Manually Reset\nRespond Flag"
                            # "Start Search Offset"
                            # "Direction"
                            # "Current Servo Angle"
                            # "delta move \nangle sum"
                            # "First Check That Robot Orientation is Still Valid"
                            n469 = local read "Position \nLock Status"() -> (w1212:bool)
                            n470 = case shown="False" w1212 {
                              tunnel: [sgl 1.0 ("y") w1215] -> w1209
                              frame False {
                                # "**Or maybe try previous direction of this servo....\ndirection would be indpedent of other servo"
                                # "Default is to move\nSame Direction as other\nServo"
                                # "No Orientation Available"
                              }
                              frame True {
                                w1216 = sgl 1.0 ("y")
                                # "Use previous position/orientation to Guess Which Direction to Move Servo"
                                # "Choose Search Direction"
                                # "\"Perpendicular \nThreshold\""
                                # "If Orientation is\n ~Perpendicular -> Start Search\n in Opposite Direction of Other"
                                # "****add 90 until orientation angle is fixed"
                                # "Fetch Last Orientation"
                                # "Convert to Rad"
                                # "Avoid Divide by 0"
                                # "-1/m"
                                # "Fetch Center Beacon Coordinates"
                                # "Calculate Normal Line to \nLast Robot Position\nfrom Center Beacon"
                                n471 = local read "Middle Beacon Coordinates"() -> (w1214:cluster{"X":sgl, "Y":sgl})
                                n472 = local read "Last Position"() -> (w1237:cluster{"X":sgl, "Y":sgl})
                                n473 = Unbundle(w1214) -> ("X"=w1234:sgl, "Y"=w1233:sgl)
                                n474 = Unbundle(w1237) -> ("X"=w1236:sgl, "Y"=w1235:sgl)
                                n475 = Subtract(x=w1235, y=w1233) -> (x-y=w1232:sgl)
                                n476 = Subtract(x=w1236, y=w1234) -> (x-y=w1230:sgl)
                                n477 = Equal To 0?(x=w1230) -> (x = 0?=w1231:bool)
                                n478 = case shown="False" w1231 {
                                tunnel: w1232 -> [w1243 _]
                                tunnel: w1230 -> [w1242 _]
                                tunnel: [w1241 1000000000000000.0] -> w1229
                                frame False {
                                n479 = Divide(x=w1243, y=w1242) -> (x/y=w1241:sgl)
                                }
                                frame True {
                                }
                                }
                                n480 = Equal To 0?(x=w1229) -> (x = 0?=w1239:bool)
                                n481 = case shown="False" w1239 {
                                tunnel: [w1245 1e-08] -> w1238
                                tunnel: w1229 -> [w1245 _]
                                frame False {
                                }
                                frame True {
                                # "Can't have infinit slope"
                                }
                                }
                                n482 = Divide(x=-1.0, y=w1238) -> (x/y=w1228:dbl)
                                n483 = Inverse Tangent(1:w1228) -> (0:w1226:dbl)
                                n484 = local read "Last Orientation"() -> (w1225:sgl)
                                n485 = expression code="(x/pi)*180.0" "radians to degrees"(w1226) -> (w1227:dbl)
                                n486 = To Single Precision Float(number=w1227) -> (single precision float=w1223:sgl)
                                n487 = Add(x=w1225, y=sgl 90.0) -> (x+y=w1222:sgl)
                                n488 = Subtract(x=w1223, y=w1222) -> (x-y=w1221:sgl)
                                n489 = Absolute Value(x=w1221) -> (abs(x)=w1220:sgl)
                                n490 = Less Or Equal?(x=w1220, y=sgl 10.0) -> (x <= y?=w1218:bool)
                                n491 = Negate(x=w1216) -> (-x=w1217:sgl)
                                n492 = Select(t=w1217, s=w1218, f=w1216) -> (s? t:f=w1215:sgl)
                              }
                            }
                            n493 = To Word Integer(number=w1209) -> (16bit integer=w1208:i16)
                            n494 = Multiply(x=w1208, y=w1207) -> (x*y=w1211:i32)
                            n495 = To Word Integer(number=w1206) -> (16bit integer=w1210:i16)
                            n496 = Add(x=w1211, y=w1210) -> (x+y=w1205:i32)
                            n497 = To Unsigned Word Integer(number=w1205) -> (unsigned 16bit integer=w1201:u16)
                          }
                        }
                        "Response\nInduced - R" <- w1147
                      }
                      frame False {
                        # "GENERIC SWEEP SEARCH"
                        # "F"
                        # "Don't Update\nKnown Track\nAngle"
                        # "Multiple New Step\nby Step SIze"
                        # "Round"
                        # "New Goal Position"
                        # "F = CCW\nT = CW"
                        # "Last Direction"
                        # "Min Step"
                        # "add 10 in case\nactual position\nis lower than GP"
                        # "Set New Step #"
                        # "Choose Direction"
                        # "Nearest step"
                        # "Adjust Actual Posiiton\n to pre-determiend steps"
                        # "Move Servo 1 \"Step\" to\nSearch"
                        n498 = Add(x=15, y=w1258) -> (x+y=w1259:i32)
                        n499 = local read "Direction - R"() -> (w1253:bool)
                        n500 = Quotient & Remainder(x=w1259, y=w1251) -> (floor(x/y)=w1263:i32)  [unwired: 1 out]
                        n501 = To Byte Integer(number=w1263) -> (8bit integer=w1254:i8)
                        n502 = Less?(x=w1254, y=1) -> (x < y?=w1266:bool)
                        n503 = case shown="False" w1266 {
                          tunnel: w1254 -> [w1277 w1285]
                          tunnel: [w1279 FALSE] -> w1261
                          tunnel: [w1278 w1285] -> w1264
                          tunnel: w1253 -> [w1276 _]
                          tunnel: w1251 -> [w1274 _]
                          frame False {
                            # "Max Step"
                            # "# of steps\nminus 1"
                            n504 = Divide(x=1024, y=w1274) -> (x/y=w1273:dbl)
                            n505 = Decrement(x=w1273) -> (x-1=w1272:dbl)
                            n506 = Greater?(x=w1277, y=w1272) -> (0:w1271:bool)
                            n507 = case shown="False" w1271 {
                              tunnel: [w1280 TRUE] -> w1279
                              tunnel: [w1281 w1282] -> w1278
                              tunnel: w1277 -> [w1281 w1282]
                              tunnel: w1276 -> [w1280 _]
                              frame False {
                                # "No Need to\nChange Direction"
                              }
                              frame True {
                                # "T"
                                # "Move CW"
                              }
                            }
                          }
                          frame True {
                            # "F"
                            # "Move CCW"
                          }
                        }
                        n508 = case shown="False" w1261 {
                          tunnel: w1264 -> [w1268 w1269]
                          tunnel: [w1267 w1270] -> w1252
                          frame False {
                            # "CCW\n+1"
                            n509 = Increment(x=w1268) -> (x+1=w1267:i8)
                          }
                          frame True {
                            # "CW\n-1"
                            n510 = Decrement(x=w1269) -> (x-1=w1270:i8)
                          }
                        }
                        "Current Step - R" <- w1252
                        n511 = Multiply(x=w1252, y=w1251) -> (x*y=w1262:u16)
                        n512 = Add(x=w1262, y=sgl 0.5) -> (x+y=w1256:sgl)
                        n513 = To Unsigned Word Integer(number=w1256) -> (unsigned 16bit integer=w1255:u16)
                      }
                    }
                  }
                }
                n514 = Increment(x=w1120) -> (x+1=w1115:i32)
              }
            }
          }
          frame True {
            # "Reset Recovery Search\nCount - Tracking Found"
            # "F"
            # "Maybe overshoot target angle?"
            # "Reset Search Cycle Count"
            # "Update Last Known Middle Beacon Angle"
            # "45 DEG MOUNT OFFSET"
            # "1024/300"
            # "Tracking logic"
            # "Reset Wait\nCount"
            # "Calculate Goal Position of Middle Angle"
            n515 = local read "Middle Beacon\nAngle - Right"() -> (w1298:sgl)
            n516 = Add(x=w1298, y=sgl 45.0) -> (x+y=w1294:sgl)
            n517 = Add(x=w1294, y=sgl 60.0) -> (x+y=w1296:sgl)
            n518 = Multiply(x=3.413333333333333, y=w1296) -> (x*y=w1299:dbl)
            n519 = Add(x=0.5, y=w1299) -> (x+y=w1291:dbl)
            n520 = To Unsigned Word Integer(number=w1291) -> (unsigned 16bit integer=w1292:u16)
          }
        }
        n521 = local read "Direction - L"() -> (w961:bool)
        n522 = case shown="False" "Angles Valid - L" {
          tunnel: w1053 -> [w1398 _]
          tunnel: [w1400 w1606] -> w1044
          tunnel: [w1399 i8 0] -> w1057
          tunnel: w1013 -> [w1383 _]
          tunnel: w1056 -> [w1397 _]
          tunnel: [w1396 u16 0] -> w1051
          tunnel: w1052 -> [w1395 _]
          tunnel: w1012 -> [w1393 _]
          tunnel: w1010 -> [w1392 _]
          tunnel: w1040 -> [w1391 _]
          tunnel: w1039 -> [w1390 _]
          tunnel: [FALSE TRUE] -> w1033
          tunnel: "Angles Valid - R" -> [w1388 _]
          tunnel: [w1387 FALSE] -> w1032
          tunnel: [w1386 FALSE] -> w1031
          tunnel: w1017 -> [w1385 _]
          tunnel: [w1384 0] -> w1019
          tunnel: w972 -> [w1382 _]
          tunnel: w971 -> [w1381 _]
          tunnel: w970 -> [w1380 _]
          tunnel: [w1379 w1599] -> w962
          tunnel: w961 -> [w1378 w1599]
          frame False {
            # "Wait Threshold Multiplier"
            # "Wait # of 'ticks' until\n1 wait cycle\n\n1 Wait Cycle is equal to\n= Servo Algorithm Cycle Time X Wait Time Factor"
            # "Searching Logic"
            n523 = Greater Or Equal?(x=w1398, y=w1383) -> (x >= y?=w1394:bool)
            n524 = case shown="True" w1394 {
              tunnel: [w1408 w1430] -> w1400
              tunnel: [w1405 i8 0] -> w1399
              tunnel: w1398 -> [w1407 _]
              tunnel: w1397 -> [w1408 w1429]
              tunnel: [w1406 w1423] -> w1396
              tunnel: w1395 -> [w1406 w1422]
              tunnel: w1393 -> [_ w1421]
              tunnel: w1392 -> [_ w1427]
              tunnel: w1391 -> [_ w1414]
              tunnel: w1390 -> [_ w1426]
              tunnel: w1388 -> [_ w1425]
              tunnel: [FALSE w1424] -> w1387
              tunnel: [FALSE w1419] -> w1386
              tunnel: w1385 -> [w1402 w1418]
              tunnel: [w1402 w1417] -> w1384
              tunnel: w1382 -> [_ w1413]
              tunnel: w1381 -> [_ w1412]
              tunnel: w1380 -> [_ w1411]
              tunnel: [w1401 w1410] -> w1379
              tunnel: w1378 -> [w1401 w1409]
              frame False {
                # "F"
                # "Current Servo Position (UINT 10)"
                # "Search Cycle Count (Don't update)"
                # "Wait Cycle Count"
                # "Increment Wait Cycle Counter, \nwait until counter is finished"
                n525 = Increment(x=w1407) -> (x+1=w1405:i8)
              }
              frame True {
                # "Reset Wait\nCount"
                # "Wait Until Start\nSearch Threshold\nto Begin Smart Search"
                # "Increment Search\n Cycle Count"
                # "Start Search Threshold..\n\nCould be added to further delay\nregular search"
                n526 = Greater Or Equal?(x=w1422, y=w1421) -> (x >= y?=w1415:bool)
                n527 = Or(x=w1415, y=w1414) -> (x .or. y?=w1416:bool)
                n528 = case shown="True" w1416 {
                  tunnel: [w1435 w1454] -> w1430
                  tunnel: w1429 -> [w1435 w1453]
                  tunnel: [w1434 w1452] -> w1428
                  tunnel: w1427 -> [_ w1451]
                  tunnel: w1426 -> [_ w1450]
                  tunnel: w1414 -> [_ w1449]
                  tunnel: w1425 -> [_ w1444]
                  tunnel: [FALSE w1448] -> w1424
                  tunnel: w1422 -> [w1434 w1447]
                  tunnel: [FALSE w1446] -> w1419
                  tunnel: w1418 -> [w1432 w1443]
                  tunnel: [w1432 w1442] -> w1417
                  tunnel: w1413 -> [_ w1441]
                  tunnel: w1412 -> [_ w1440]
                  tunnel: w1411 -> [_ _]
                  tunnel: [w1431 w1438] -> w1410
                  tunnel: w1409 -> [w1431 w1437]
                  frame False {
                    # "F"
                    # "Do Nothing, \nwait until Search Count is Above Threshold"
                  }
                  frame True {
                    # "Or if Other Servo\nHas Trackin Info"
                    # "Only Attempt\nSmart Search \nUntil This count"
                    # "Current Servo Position"
                    n529 = Less?(x=w1447, y=w1441) -> (x < y?=w1445:bool)
                    n530 = Compound Arithmetic op=OR(w1445, w1444) -> (w1439:bool)
                    n531 = case shown="True" w1439 {
                      tunnel: [w1468 w1569] -> w1454
                      tunnel: w1453 -> [w1464 w1571]
                      tunnel: [w1465 w1564] -> w1452
                      tunnel: w1451 -> [w1460 w1566]
                      tunnel: w1449 -> [w1457 _]
                      tunnel: w1450 -> [w1469 _]
                      tunnel: w1447 -> [w1465 w1564]
                      tunnel: w1444 -> [w1467 _]
                      tunnel: [w1466 FALSE] -> w1448
                      tunnel: [w1463 FALSE] -> w1446
                      tunnel: w1443 -> [w1462 w1562]
                      tunnel: [w1461 w1562] -> w1442
                      tunnel: w1440 -> [w1456 _]
                      tunnel: [w1455 w1560] -> w1438
                      tunnel: w1437 -> [w1455 w1559]
                      frame True {
                        # "SMART SEARCH"
                        # "******************************\ninstead of limiting when reactive\ncan occur... maybe just have this number\nset the preference for which\nrecovery technique to use"
                        # "Search Must Be\nLess than this to Attempt\nReactive Recovery Search\n\nWill Attempt Recovery Search\nAfter This"
                        # "Search Goal\nPosition"
                        # "Move Respond - L"
                        # "Check if other\nservo moved\n& Search < 3"
                        # "Since first time searching \nsince previously tracking,\n if this servo hasn't responded to other's last movement\nUse it to Predict where to begin Search"
                        n532 = Less?(x=w1465, y=w1456) -> (x < y?=w1459:bool)
                        n533 = And(x=w1457, y=w1459) -> (x .and. y?=w1458:bool)
                        n534 = case shown="False" w1458 {
                          tunnel: w1464 -> [_ w1518]
                          tunnel: w1469 -> [_ w1519]
                          tunnel: [w1476 w1513] -> w1468
                          tunnel: w1467 -> [w1471 _]
                          tunnel: [w1477 FALSE] -> w1466
                          tunnel: w1464 -> [w1475 _]
                          tunnel: [FALSE TRUE] -> w1463
                          tunnel: w1462 -> [w1473 w1514]
                          tunnel: [w1472 w1514] -> w1461
                          tunnel: w1460 -> [w1470 _]
                          frame False {
                            # "And Right Servo"
                            # "Right Servo Track \nAngle Valid?"
                            # "F"
                            # "Reactive Search Using Other Servo Feedback Not Available...\nAttempt Recovery Search if Other Servo is Tracking"
                            n535 = case shown="True" w1471 {
                              tunnel: [FALSE TRUE] -> w1477
                              tunnel: [w1478 w1482] -> w1476
                              tunnel: w1475 -> [w1478 w1487]
                              tunnel: w1473 -> [w1479 w1485]
                              tunnel: [w1479 w1484] -> w1472
                              tunnel: w1470 -> [_ w1481]
                              frame False {
                                # "No Info Available.... do nothin for now... maybe move a little"
                                # "F"
                              }
                              frame True {
                                # "Recover Search\nCount"
                                # "****************\n*************"
                                # "If 0, Set GP to parallel\n-increment count\nIf >0, Pan CW by step size/2\nIf > 5, reset count\n\nreset count in Track case too"
                                # "Check # of Times\nThis Case Has Been\nEntered"
                                n536 = Greater Than 0?(x=w1485) -> (x > 0?=w1486:bool)
                                n537 = case shown="False" w1486 {
                                tunnel: [w1490 w1504] -> w1482
                                tunnel: w1487 -> [_ w1505]
                                tunnel: w1485 -> [w1488 w1506]
                                tunnel: [w1489 w1507] -> w1484
                                tunnel: w1481 -> [_ w1502]
                                frame False {
                                # "Move Servo Parallel to Other Servo"
                                # "First Attempt at Recovery Search"
                                # "45 DEG MOUNT OFFSET"
                                # "1024/300"
                                n538 = local read "Middle Beacon\nAngle - Right"() -> (w1492:sgl)
                                n539 = Increment(x=w1488) -> (x+1=w1489:i32)
                                n540 = Subtract(x=w1492, y=sgl 45.0) -> (x-y=w1494:sgl)
                                n541 = Add(x=w1494, y=sgl 60.0) -> (x+y=w1496:sgl)
                                n542 = Multiply(x=3.413333333333333, y=w1496) -> (x*y=w1498:dbl)
                                n543 = Add(x=0.5, y=w1498) -> (x+y=w1491:dbl)
                                n544 = To Unsigned Word Integer(number=w1491) -> (unsigned 16bit integer=w1490:u16)
                                }
                                frame True {
                                # "sTEP siZE\nfine factor"
                                # "Attempt to Pan in Steps Towards other Servo"
                                # "Could be same or function of \nregular search step size"
                                # "CW = subtract"
                                # "MAKE SURE ADDING/SUBTRACTING\nTO RIGHT DIRECTION"
                                # "Search Count Greater Than 0"
                                n545 = Greater Or Equal?(x=w1506, y=u16 10) -> (x >= y?=w1508:bool)
                                n546 = case shown="True" w1508 {
                                tunnel: [w1510 u16 0 ("y")] -> w1507
                                tunnel: w1506 -> [w1511 _]
                                frame False {
                                # "Increment Count"
                                # "Continue to Pan until Limit Reached"
                                n547 = Increment(x=w1511) -> (x+1=w1510:i32)
                                }
                                frame True {
                                # "Count (pan attempts) limit reached\n\nReset Count"
                                }
                                }
                                n548 = Divide(x=w1502, y=u16 3) -> (x/y=w1501:dbl)
                                n549 = To Unsigned Word Integer(number=w1501) -> (unsigned 16bit integer=w1500:u16)
                                n550 = Subtract(x=w1505, y=w1500) -> (x-y=w1504:u16)
                                }
                                }
                              }
                            }
                          }
                          frame True {
                            # "Reactive Recovery Search using Other Servo Elapsed Movements"
                            # "Other Servo Has Moved - Use History of Other Servo to Estimate Search Start Position"
                            # "** check this"
                            # "Manually Reset\nRespond Flag"
                            # "Start Search Offset"
                            # "Direction"
                            # "Current Servo Angle"
                            # "delta move \nangle sum"
                            # "First Check That Robot Orientation is Still Valid"
                            n551 = local read "Position \nLock Status"() -> (w1524:bool)
                            n552 = case shown="True" w1524 {
                              tunnel: [sgl 1.0 ("y") w1526] -> w1521
                              frame False {
                                # "**Or maybe try previous direction of this servo....\ndirection would be indpedent of other servo"
                                # "Default is to move\nSame Direction as other\nServo"
                                # "No Orientation Available"
                              }
                              frame True {
                                w1527 = sgl 1.0 ("y")
                                # "Use previous position/orientation to Guess Which Direction to Move Servo"
                                # "Choose Search Direction"
                                # "\"Perpendicular \nThreshold\""
                                # "If Orientation is\n ~Perpendicular -> Start Search\n in Opposite Direction of Other"
                                # "****add 90 until orientation angle is fixed"
                                # "Fetch Last Orientation"
                                # "Convert to Rad"
                                # "Avoid Divide by 0"
                                # "-1/m"
                                # "Fetch Center Beacon Coordinates"
                                # "Calculate Normal Line to \nLast Robot Position\nfrom Center Beacon"
                                n553 = local read "Last Position"() -> (w1548:cluster{"X":sgl, "Y":sgl})
                                n554 = Unbundle("Middle Beacon Coordinates") -> ("X"=w1545:sgl, "Y"=w1544:sgl)
                                n555 = Unbundle(w1548) -> ("X"=w1547:sgl, "Y"=w1546:sgl)
                                n556 = Subtract(x=w1546, y=w1544) -> (x-y=w1543:sgl)
                                n557 = Subtract(x=w1547, y=w1545) -> (x-y=w1541:sgl)
                                n558 = Equal To 0?(x=w1541) -> (x = 0?=w1542:bool)
                                n559 = case shown="False" w1542 {
                                tunnel: w1543 -> [w1555 _]
                                tunnel: w1541 -> [w1554 _]
                                tunnel: [w1553 1000000000000000.0] -> w1540
                                frame False {
                                n560 = Divide(x=w1555, y=w1554) -> (x/y=w1553:sgl)
                                }
                                frame True {
                                }
                                }
                                n561 = Equal To 0?(x=w1540) -> (x = 0?=w1550:bool)
                                n562 = case shown="False" w1550 {
                                tunnel: [w1557 1e-08] -> w1549
                                tunnel: w1540 -> [w1557 _]
                                frame False {
                                }
                                frame True {
                                # "Can't have infinit slope"
                                }
                                }
                                n563 = Divide(x=-1.0, y=w1549) -> (x/y=w1539:dbl)
                                n564 = Inverse Tangent(1:w1539) -> (0:w1537:dbl)
                                n565 = local read "Last Orientation"() -> (w1536:sgl)
                                n566 = expression code="(x/pi)*180.0" "radians to degrees"(w1537) -> (w1538:dbl)
                                n567 = To Single Precision Float(number=w1538) -> (single precision float=w1534:sgl)
                                n568 = Add(x=w1536, y=sgl 90.0) -> (x+y=w1533:sgl)
                                n569 = Subtract(x=w1534, y=w1533) -> (x-y=w1532:sgl)
                                n570 = Absolute Value(x=w1532) -> (abs(x)=w1531:sgl)
                                n571 = Less Or Equal?(x=w1531, y=sgl 10.0) -> (x <= y?=w1529:bool)
                                n572 = Negate(x=w1527) -> (-x=w1528:sgl)
                                n573 = Select(t=w1528, s=w1529, f=w1527) -> (s? t:f=w1526:sgl)
                              }
                            }
                            n574 = To Word Integer(number=w1521) -> (16bit integer=w1520:i16)
                            n575 = Multiply(x=w1520, y=w1519) -> (x*y=w1523:i32)
                            n576 = To Word Integer(number=w1518) -> (16bit integer=w1522:i16)
                            n577 = Add(x=w1523, y=w1522) -> (x+y=w1517:i32)
                            n578 = To Unsigned Word Integer(number=w1517) -> (unsigned 16bit integer=w1513:u16)
                          }
                        }
                        "Response\nInduced - L" <- w1457
                      }
                      frame False {
                        # "F"
                        # "GENERIC SWEEP SEARCH"
                        # "Don't Update\nKnown Track\nAngle"
                        # "Multiple New Step\nby Step SIze"
                        # "Round"
                        # "New Goal Position"
                        # "F = CCW\nT = CW"
                        # "Last Direction"
                        # "Min Step"
                        # "add 10 in case\nactual position\nis lower than GP"
                        # "Set New Step #"
                        # "Choose Direction"
                        # "Nearest step"
                        # "Adjust Actual Posiiton\n to pre-determiend steps"
                        # "Move Servo 1 \"Step\" to\nSearch"
                        n579 = Add(x=5, y=w1571) -> (x+y=w1572:i32)
                        n580 = Quotient & Remainder(x=w1572, y=w1566) -> (floor(x/y)=w1575:i32)  [unwired: 1 out]
                        n581 = To Byte Integer(number=w1575) -> (8bit integer=w1568:i8)
                        n582 = Less?(x=w1568, y=1) -> (x < y?=w1578:bool)
                        n583 = case shown="False" w1578 {
                          tunnel: w1568 -> [w1590 w1598]
                          tunnel: [w1592 FALSE] -> w1560
                          tunnel: [w1591 w1598] -> w1576
                          tunnel: w1559 -> [w1589 _]
                          tunnel: w1566 -> [w1587 _]
                          frame False {
                            # "Max Step"
                            # "# of steps\nminus 1"
                            n584 = Divide(x=1024, y=w1587) -> (x/y=w1584:dbl)
                            n585 = Decrement(x=w1584) -> (x-1=w1583:dbl)
                            n586 = To Unsigned Byte Integer(number=w1583) -> (unsigned 8bit integer=w1585:u8)
                            n587 = Greater Or Equal?(x=w1590, y=w1585) -> (x >= y?=w1586:bool)
                            n588 = case shown="True" w1586 {
                              tunnel: [w1593 TRUE] -> w1592
                              tunnel: [w1594 w1595] -> w1591
                              tunnel: w1590 -> [w1594 w1595]
                              tunnel: w1589 -> [w1593 _]
                              frame False {
                                # "No Need to\nChange Direction"
                              }
                              frame True {
                                # "T"
                                # "Move CW"
                              }
                            }
                          }
                          frame True {
                            # "F"
                            # "Move CCW"
                          }
                        }
                        n589 = case shown="False" w1560 {
                          tunnel: w1576 -> [w1580 w1581]
                          tunnel: [w1579 w1582] -> w1567
                          frame False {
                            # "CCW\n+1"
                            n590 = Increment(x=w1580) -> (x+1=w1579:i8)
                          }
                          frame True {
                            # "CW\n-1"
                            n591 = Decrement(x=w1581) -> (x-1=w1582:i8)
                          }
                        }
                        "Current Step - L" <- w1567
                        n592 = Multiply(x=w1567, y=w1566) -> (x*y=w1574:u16)
                        n593 = Add(x=w1574, y=sgl 0.5) -> (x+y=w1570:sgl)
                        n594 = To Unsigned Word Integer(number=w1570) -> (unsigned 16bit integer=w1569:u16)
                      }
                    }
                  }
                }
                n595 = Increment(x=w1428) -> (x+1=w1423:i32)
              }
            }
          }
          frame True {
            # "Reset Recovery Search\nCount - Tracking Found"
            # "F"
            # "Maybe overshoot target angle?"
            # "Reset Search Cycle Count"
            # "Update Last Known Middle Beacon Angle"
            # "45 DEG MOUNT OFFSET"
            # "1024/300"
            # "Tracking logic"
            # "Reset Wait\nCount"
            # "Calculate Goal Position of Middle Angle"
            n596 = local read "Middle Beacon\nAngle - Left"() -> (w1612:sgl)
            n597 = Subtract(x=w1612, y=sgl 45.0) -> (x-y=w1608:sgl)
            n598 = Add(x=w1608, y=sgl 60.0) -> (x+y=w1610:sgl)
            n599 = Multiply(x=3.413333333333333, y=w1610) -> (x*y=w1613:dbl)
            n600 = Add(x=0.5, y=w1613) -> (x+y=w1605:dbl)
            n601 = To Unsigned Word Integer(number=w1605) -> (unsigned 16bit integer=w1606:u16)
          }
        }
        n602 = Less?(x=w1044, y=w1043) -> (x < y?=w1045:bool)
        n603 = Less?(x=w992, y=w998) -> (x < y?=w999:bool)
        n604 = Select(t=w1044, s=w1045, f=w1043) -> (s? t:f=w1036:u16)
        n605 = Select(t=w992, s=w999, f=w998) -> (s? t:f=w989:u16)
        n606 = To Word Integer(number=w1036) -> (16bit integer=w1055:i16)
        n607 = To Word Integer(number=w1056) -> (16bit integer=w1054:i16)
        n608 = Subtract(x=w1055, y=w1054) -> (x-y=w1038:i16)
        n609 = To Word Integer(number=w989) -> (16bit integer=w1006:i16)
        n610 = To Word Integer(number=w976) -> (16bit integer=w1005:i16)
        n611 = Absolute Value(x=w1038) -> (abs(x)=w1046:i16)
        n612 = Subtract(x=w1006, y=w1005) -> (x-y=w996:i16)
        n613 = Absolute Value(x=w996) -> (abs(x)=w1000:i16)
        n614 = To Long Integer(number=w1036) -> (32bit integer=w1049:i32)
        n615 = To Long Integer(number=w1035) -> (32bit integer=w1050:i32)
        n616 = Greater?(x=w1046, y=w975) -> (0:w1047:bool)
        n617 = Subtract(x=w1049, y=w1050) -> (x-y=w1030:i32)
        n618 = To Long Integer(number=w989) -> (32bit integer=w1003:i32)
        n619 = To Long Integer(number=w991) -> (32bit integer=w1004:i32)
        n620 = Greater?(x=w1000, y=w975) -> (0:w1001:bool)
        n621 = Subtract(x=w1003, y=w1004) -> (x-y=w993:i32)
        n622 = Not Equal To 0?(x=w1030) -> (x != 0?=w1042:bool)
        n623 = Less?(x=w1046, y=w974) -> (x < y?=w1048:bool)
        n624 = Less Than 0?(x=w1038) -> ()  [unwired: 1 out]
        n625 = Not Equal To 0?(x=w993) -> (x != 0?=w997:bool)
        n626 = Less?(x=w1000, y=w974) -> (x < y?=w1002:bool)
        n627 = Less Than 0?(x=w996) -> (x < 0?=w994:bool)
        n628 = Compound Arithmetic op=AND(w1042, w1048, w1047) -> (w963:bool)
        n629 = Compound Arithmetic op=AND(w997, w1002, w1001) -> (w990:bool)
        n630 = case shown="True" w1032 {
          selector: w1032 -> [_ w1373]
          tunnel: w962 -> [w1372 _]
          tunnel: [w1372 w1373] -> w969
          frame False {
            # "CCW"
          }
          frame True {
            # "CW"
          }
        }
        n631 = case shown="True" w977 {
          selector: w977 -> [_ w1070]
          tunnel: w994 -> [w1068 _]
          tunnel: [w1068 w1069] -> w967
          frame False {
            # "CW"
          }
          frame True {
            # "CCW"
            n632 = Not(x=w1070) -> (.not. x?=w1069:bool)
          }
        }
        n633 = And(x=w1033, y=w963) -> (x .and. y?=w1037:bool)
        n634 = And(x=w986, y=w990) -> (x .and. y?=w995:bool)
        n635 = case shown="True" w1037 {
          tunnel: w1036 -> [_ w1377]
          tunnel: [w1375 w1377] -> w1034
          tunnel: w1035 -> [w1375 _]
          tunnel: w1030 -> [_ w1376]
          tunnel: [0 w1376] -> w1029
          frame False {
            # "no delta bc no movement"
            # "Use Old Value for Tracking\nAngle"
          }
          frame True {
            # "Use this delta"
            # "New Tracking Position"
          }
        }
        "Last Known\nTracking Position - L" <- w1034
        n636 = case shown="False" w964 {
          selector: w964 -> [_ w1062]
          tunnel: [w1060 w1061] -> w968
          tunnel: w969 -> [w1060 _]
          frame False {
          }
          frame True {
            n637 = Not(x=w1062) -> (.not. x?=w1061:bool)
          }
        }
        n638 = case shown="True" w964 {
          selector: w964 -> [_ w1059]
          tunnel: [w1058 w1059] -> w966
          tunnel: w967 -> [w1058 _]
          frame False {
          }
          frame True {
          }
        }
        n639 = case shown="True" w995 {
          tunnel: w989 -> [_ w1074]
          tunnel: [w1072 w1074] -> w988
          tunnel: w991 -> [w1072 _]
          tunnel: w993 -> [_ w1073]
          tunnel: [0 w1073] -> w987
          frame False {
            # "no delta bc no movement"
            # "Use Old Value for Tracking\nAngle"
          }
          frame True {
            # "Use this delta"
            # "New Tracking Position"
          }
        }
        "Last Known\nTracking Position - R" <- w988
        n640 = flat-sequence {
          tunnel: w963 -> [w1303]
          tunnel: w990 -> [w1302]
          tunnel: w966 -> [w1307]
          tunnel: w1036 -> [w1306]
          tunnel: w989 -> [w1305]
          tunnel: w968 -> [w1304]
          tunnel: [w1303] -> w1022
          tunnel: [w1302] -> w1018
          tunnel: w1022 -> [w1315]
          tunnel: [w1314] -> w1021
          tunnel: [w1313] -> w1020
          tunnel: w1018 -> [w1312]
          frame #0 {
            # "Only Update GP if Moving Servo"
            n641 = case shown="True" w1303 {
              tunnel: w1306 -> [_ w1311]
              tunnel: w1304 -> [_ w1310]
              frame False {
              }
              frame True {
                # "New Direction"
                # "Update Direction"
                # "Update Goal Position"
                n642 = local write "Servo Goal Position\n - Left"(w1311) -> ()
                "Direction - L" <- w1310
              }
            }
            n643 = case shown="True" w1302 {
              tunnel: w1305 -> [_ w1309]
              tunnel: w1307 -> [_ w1308]
              frame False {
              }
              frame True {
                # "New Direction"
                # "Update Goal Position"
                # "Update Direction"
                n644 = local write "Servo Goal Position\n - Right"(w1309) -> ()
                "Direction - R" <- w1308
              }
            }
          }
          frame #1 {
            # "Allow Comm Process to Take Down the Flag\nOnly Raise if not already in motion"
            n645 = local read "Servo Moving - R"() -> (w1320:bool)
            n646 = local read "Servo Moving - L"() -> (w1317:bool)
            n647 = local read "Move Servo - L"() -> (w1316:bool)
            n648 = local read "Move Servo - R"() -> (w1323:bool)
            n649 = Not(x=w1320) -> (.not. x?=w1322:bool)
            n650 = Not(x=w1317) -> (.not. x?=w1319:bool)
            n651 = And(x=w1312, y=w1322) -> (x .and. y?=w1321:bool)
            n652 = And(x=w1315, y=w1319) -> (x .and. y?=w1318:bool)
            n653 = case shown="True" w1321 {
              selector: w1321 -> [_ w1325]
              tunnel: [w1324 w1325] -> w1313
              tunnel: w1323 -> [w1324 _]
              frame False {
              }
              frame True {
              }
            }
            n654 = case shown="True" w1318 {
              selector: w1318 -> [_ w1327]
              tunnel: [w1326 w1327] -> w1314
              tunnel: w1316 -> [w1326 _]
              frame False {
              }
              frame True {
              }
            }
            n655 = local write "Move Servo - R"(w1313) -> ()
            n656 = local write "Move Servo - L"(w1314) -> ()
          }
        }
        n657 = And(x=w1033, y=w1021) -> (x .and. y?=w1026:bool)
        n658 = And(x=w1020, y=w986) -> (x .and. y?=w1025:bool)
        n659 = Exclusive Or(1:w1025, 2:w1026) -> (0:w1028:bool)
        n660 = And(x=w1033, y=w986) -> (x .and. y?=w1027:bool)
        n661 = case shown="True" w1028 {
          tunnel: [w1338 w1359] -> w982
          tunnel: [w1339 w1358] -> w1024
          tunnel: w987 -> [_ w1362]
          tunnel: w1039 -> [w1336 w1363]
          tunnel: w983 -> [w1334 w1361]
          tunnel: [w1337 w1349] -> w1023
          tunnel: [w1335 w1348] -> w981
          tunnel: w1029 -> [_ w1360]
          tunnel: w1027 -> [w1333 _]
          tunnel: w1026 -> [_ w1359]
          tunnel: w1025 -> [_ w1358]
          frame False {
            n662 = case shown="False" w1333 {
              tunnel: [w1343 w1345] -> w1339
              tunnel: [w1342 w1345] -> w1338
              tunnel: [w1341 w1344] -> w1337
              tunnel: w1336 -> [w1341 _]
              tunnel: [w1340 w1344] -> w1335
              tunnel: w1334 -> [w1340 _]
              frame False {
                # "No Movement\nRetain All Values"
                n663 = local read "Move Respond - L"() -> (w1343:bool)
                n664 = local read "Move Respond - R"() -> (w1342:bool)
              }
              frame True {
                w1344 = i16 0
                w1345 = FALSE
                # "Reset Delta Move sum\nfor both"
                # "F"
                # "Both Moved,\nMake Flags False"
              }
            }
          }
          frame True {
            w1355 = 200 ("y")
            w1346 = -200 ("y")
            # "Add/Clear Sum for \nServo That didn't move"
            # "Update Moving Servo's  Delta Position"
            # "if one Servo Moves, other should \nmove too eventually,\nUsed in Search Process"
            # "Only 1 Servo is Moving Due to Tracking --> Update delta move sum"
            n665 = case shown="True" w1358 {
              tunnel: w1363 -> [_ w1371]
              tunnel: w1362 -> [_ w1370]
              tunnel: [i16 0 w1369] -> w1356
              frame False {
              }
              frame True {
                n666 = Add(x=w1371, y=w1370) -> (x+y=w1369:i32)
              }
            }
            n667 = case shown="True" w1359 {
              tunnel: w1361 -> [_ w1367]
              tunnel: w1360 -> [_ w1366]
              tunnel: [i16 0 w1365] -> w1353
              frame False {
              }
              frame True {
                n668 = Add(x=w1367, y=w1366) -> (x+y=w1365:i32)
              }
            }
            n669 = Greater?(x=w1356, y=w1355) -> (0:w1357:bool)
            n670 = Greater?(x=w1353, y=w1355) -> (0:w1354:bool)
            n671 = Select(t=w1355, s=w1354, f=w1353) -> (s? t:f=w1350:i32)
            n672 = Select(t=w1355, s=w1357, f=w1356) -> (s? t:f=w1351:i32)
            n673 = Greater?(x=w1351, y=w1346) -> (0:w1347:bool)
            n674 = Greater?(x=w1350, y=w1346) -> (0:w1352:bool)
            n675 = Select(t=w1350, s=w1352, f=w1346) -> (s? t:f=w1348:i32)
            n676 = Select(t=w1351, s=w1347, f=w1346) -> (s? t:f=w1349:i32)
          }
        }
        n677 = case shown="True" w973 {
          selector: w973 -> [_ w1067]
          tunnel: [w1064 w1066] -> w980
          tunnel: [w1063 i16 0] -> w979
          tunnel: w982 -> [w1064 _]
          tunnel: w981 -> [w1063 _]
          frame False {
          }
          frame True {
            n678 = Not(x=w1067) -> (.not. x?=w1066:bool)
          }
        }
        "Move Respond - R" <- w980
        "deltaMoveServo\n- R" <- w979
        n679 = case shown="True" w1031 {
          selector: w1031 -> [_ w1332]
          tunnel: [w1329 w1331] -> w1041
          tunnel: [w1328 i16 0] -> w978
          tunnel: w1024 -> [w1329 _]
          tunnel: w1023 -> [w1328 _]
          frame False {
          }
          frame True {
            n680 = Not(x=w1332) -> (.not. x?=w1331:bool)
          }
        }
        "Move Respond - L" <- w1041
        "deltaMoveServo\n- L" <- w978
        "Wait Cycle Count - L" <- w1053
        "Wait Count - R" <- w1015
        "Recovery Search Count L" <- w1017
        "Recovery Search Count R" <- w1008
      }
    }
    n681 = call "Wait"("Count(mSec)"="Servo Algorithm\nCycle Time(ms)") -> ()  [unwired: 1 out]
    n682 = local read "Direction - L"() -> (w902:bool)
    n683 = local read "Direction - R"() -> (w901:bool)
    "Search Count - L" <- w880
    "Search Count - R" <- w876
  }
  n684 = flat-sequence {
    tunnel: [w1618] -> w36
    tunnel: [w1617] -> w35
    tunnel: [w1622] -> w34
    tunnel: ["Left Servo\nID"] -> w14
    tunnel: ["Right Servo\nID"] -> w13
    tunnel: ["Compliance Slope"] -> w11
    tunnel: [w1662] -> w33
    tunnel: [w1661] -> w32
    tunnel: w36 -> [w1660]
    tunnel: w35 -> [w1659]
    tunnel: w34 -> [w1658]
    tunnel: w14 -> [w1656]
    tunnel: w13 -> [w1655]
    tunnel: w11 -> [w1654]
    tunnel: w33 -> [w1937]
    tunnel: w32 -> [w1936]
    frame #0 {
      # "BAUD RATE"
      # "Initialize UART and DIO"
      n685 = call-poly "VISA Configure Serial Port"("VISA resource name"=refnum<visa-resource-name> "ASRL1::INSTR", "Enable Termination\nChar (T)"=FALSE ("Enable Termination\nChar (T)"), "baud rate (9600)"=u32 115200) -> ("VISA resource name out"=w1618:refnum<visa-resource-name>)  [unwired: 11 in, 1 out]
      n686 = call <vilib>:"Smart Open.vi"("Channel Names"=tag[] ["A/DIO2"]) -> ("DIO Ref Out"=w1617:T4)  [unwired: 9 in, 1 out]
      n687 = flat-sequence {
        tunnel: w1618 -> [w1630]
        tunnel: w1617 -> [w1629]
        tunnel: "Left Servo\nID" -> [w1631]
        tunnel: [w1628] -> w1619
        tunnel: "Compliance Slope" -> [w1627]
        tunnel: "Right Servo\nID" -> [w1644]
        tunnel: w1619 -> [w1643]
        tunnel: "Compliance Slope" -> [w1642]
        tunnel: w1618 -> [w1641]
        tunnel: w1617 -> [w1640]
        frame #0 {
          w1628 = 3
          n688 = while {
            tunnel: w1628 -> [w1637]
            tunnel: w1630 -> [w1635]
            tunnel: w1629 -> [w1634]
            tunnel: w1631 -> [w1633]
            tunnel: w1627 -> [w1632]
            i -> [w1638]
            stop <- w1636 stop-if-true
            n689 = call "Set_Compliance_Slope_R2.vi"("Compliance Slope"=w1632, "DIO Ref Out"=w1634, "VISA resource name"=w1635, "Servo ID"=w1633) -> ()  [unwired: 6 in, 2 out]
            n690 = Increment(x=w1638) -> (x+1=w1639:i32)
            n691 = Greater Or Equal?(x=w1639, y=w1637) -> (x >= y?=w1636:bool)
          }
        }
        frame #1 {
          n692 = while {
            tunnel: w1643 -> [w1650]
            tunnel: w1644 -> [w1648]
            tunnel: w1641 -> [w1647]
            tunnel: w1640 -> [w1646]
            tunnel: w1642 -> [w1645]
            i -> [w1651]
            stop <- w1649 stop-if-true
            n693 = call "Set_Compliance_Slope_R2.vi"("Compliance Slope"=w1645, "DIO Ref Out"=w1646, "VISA resource name"=w1647, "Servo ID"=w1648) -> ()  [unwired: 6 in, 2 out]
            n694 = Increment(x=w1651) -> (x+1=w1652:i32)
            n695 = Greater Or Equal?(x=w1652, y=w1650) -> (x >= y?=w1649:bool)
          }
        }
      }
      n696 = call "Tick Count"() -> ("Tick Count(uSec)"=w1622:u32)
    }
    frame #1 {
      # "Service Count"
      n697 = while {
        shift-right: [w1664] -> _
        shift-left: w1658 -> [w1684]
        tunnel: "Max Write\nTx Attempts" -> [w1679]
        tunnel: "Max Read\nTx Attempts" -> [w1678]
        shift-right: [w1674] -> w1662
        shift-left: w1660 -> [w1677]
        shift-right: [w1673] -> w1661
        shift-left: w1659 -> [w1676]
        tunnel: w1656 -> [w1669]
        tunnel: w1655 -> [w1668]
        tunnel: w1654 -> [w1667]
        shift-right: [w1665] -> _
        shift-left: u16 0 -> [w1666]
        stop <- "close comms" stop-if-true
        # "Loop Timer"
        n698 = local read "MANUAL SERVO \nCONTROL ENABLE"() -> (w1670:bool)
        n699 = local read "SERVO ENABLE"() -> (w1671:bool)
        n700 = call "Tick Count2"() -> ("Tick Count(uSec)"=w1664:u32)
        n701 = Subtract(x=w1664, y=w1684) -> (x-y=w1683:u32)
        n702 = call "Wait4"("Count(mSec)"="Servo Comm\nLoop Time (ms)") -> ()  [unwired: 1 out]
        n703 = Divide(x=w1683, y=u32 1000) -> (x/y=→"dT - Comm Loop":dbl)
        n704 = Exclusive Or(1:w1670, 2:w1671) -> (0:w1672:bool)
        n705 = case shown="True" w1672 {
          tunnel: w1679 -> [_ w1692]
          tunnel: w1678 -> [_ w1724]
          tunnel: w1677 -> [w1687 w1704]
          tunnel: w1676 -> [w1686 w1717]
          tunnel: [w1687 w1689] -> w1674
          tunnel: [w1686 w1688] -> w1673
          tunnel: w1669 -> [_ w1695]
          tunnel: w1668 -> [_ w1694]
          tunnel: w1667 -> [_ w1693]
          tunnel: w1666 -> [_ w1691]
          tunnel: [u16 100 w1690] -> w1665
          frame False {
            # "Restart at same value\nUsed to Periodically update \nCompliance Slope"
          }
          frame True {
            n706 = flat-sequence {
              tunnel: [w1730] -> w1728
              tunnel: [w1731] -> w1727
              tunnel: [w1729] -> w1726
              tunnel: w1724 -> [w1732]
              tunnel: [w1734] -> w1715
              tunnel: [w1733] -> w1713
              tunnel: w1704 -> [w1734]
              tunnel: w1717 -> [w1733]
              tunnel: w1695 -> [w1729]
              tunnel: w1728 -> [w1752]
              tunnel: w1727 -> [w1753]
              tunnel: w1726 -> [w1751]
              tunnel: [w1751] -> w1725
              tunnel: [w1750] -> w1718
              tunnel: [w1749] -> w1716
              tunnel: w1715 -> [w1749]
              tunnel: [w1748] -> w1714
              tunnel: w1713 -> [w1748]
              tunnel: w1725 -> [w1774]
              tunnel: w1692 -> [w1773]
              tunnel: w1718 -> [w1768]
              tunnel: w1716 -> [w1770]
              tunnel: w1714 -> [w1769]
              tunnel: [w1770] -> w1711
              tunnel: [w1769] -> w1709
              tunnel: [w1807] -> w1712
              tunnel: w1711 -> [w1807]
              tunnel: [w1806] -> w1710
              tunnel: w1709 -> [w1806]
              tunnel: ["Servo Comm\nWait Time - (ms)"] -> w1700
              tunnel: w1724 -> [w1814]
              tunnel: [w1813] -> w1723
              tunnel: [w1812] -> w1722
              tunnel: [w1808] -> w1720
              tunnel: w1712 -> [w1811]
              tunnel: w1710 -> [w1810]
              tunnel: [w1811] -> w1708
              tunnel: [w1810] -> w1705
              tunnel: [w1809] -> w1701
              tunnel: w1700 -> [w1809]
              tunnel: w1694 -> [w1808]
              tunnel: w1723 -> [w1834]
              tunnel: w1722 -> [w1833]
              tunnel: [w1832] -> w1721
              tunnel: w1720 -> [w1832]
              tunnel: [w1831] -> w1719
              tunnel: w1708 -> [w1830]
              tunnel: [w1830] -> w1707
              tunnel: [w1829] -> w1706
              tunnel: w1705 -> [w1829]
              tunnel: w1701 -> [w1828]
              tunnel: [w1828] -> w1699
              tunnel: w1721 -> [w1856]
              tunnel: w1719 -> [w1854]
              tunnel: w1692 -> [w1855]
              tunnel: w1707 -> [w1853]
              tunnel: w1706 -> [w1852]
              tunnel: [w1853] -> w1703
              tunnel: [w1852] -> w1702
              tunnel: w1699 -> [w1849]
              tunnel: [w1849] -> w1698
              tunnel: w1703 -> [w1889]
              tunnel: w1702 -> [w1888]
              tunnel: w1698 -> [w1887]
              tunnel: [w1889] -> w1697
              tunnel: [w1888] -> w1696
              tunnel: w1697 -> [w1893]
              tunnel: w1696 -> [w1892]
              tunnel: w1695 -> [w1898]
              tunnel: w1694 -> [w1897]
              tunnel: w1693 -> [w1896]
              tunnel: w1691 -> [w1891]
              tunnel: w1692 -> [w1895]
              tunnel: [w1894] -> w1690
              tunnel: [w1893] -> w1689
              tunnel: [w1892] -> w1688
              frame #0 {
                n707 = while {
                  tunnel: [w1747] -> w1730
                  tunnel: w1729 -> [w1746]
                  tunnel: [w1739] -> w1731
                  tunnel: w1732 -> [w1737]
                  tunnel: w1734 -> [w1736]
                  tunnel: w1733 -> [w1735]
                  i -> [w1738]
                  stop <- w1740 stop-if-true
                  # "Attemp to Read Until\nMax Read Tx Attemps Limit"
                  n708 = call "ReadServo_R3.vi"("DIO Ref In"=w1735, "VISA resource name out"=w1736, "Servo ID"=w1746) -> ("Error"=w1743:u8, "Valid Checksum"=w1744:bool, "Current Position"=w1747:u64)  [unwired: 6 in]
                  n709 = Increment(x=w1738) -> (x+1=w1741:i32)
                  n710 = Equal To 0?(x=w1743) -> (x = 0?=w1745:bool)
                  n711 = Greater Or Equal?(x=w1741, y=w1737) -> (x >= y?=w1742:bool)
                  n712 = And(x=w1744, y=w1745) -> (x .and. y?=w1739:bool)
                  n713 = Or(x=w1739, y=w1742) -> (x .or. y?=w1740:bool)
                }
              }
              frame #1 {
                # "Read Position First"
                n714 = local read "Servo Goal Position\n - Left"() -> (w1750:u16)
                n715 = case shown="True" w1753 {
                  tunnel: w1752 -> [_ w1758]
                  tunnel: w1750 -> [_ w1756]
                  frame False {
                  }
                  frame True {
                    # "Convert Received Position to Angle Relative to Robot"
                    # "45 DEG MOUNT OFFSET"
                    # "1024/300"
                    n716 = local write "Current L (10bit)"(w1758) -> ()
                    n717 = To Word Integer(number=w1758) -> (16bit integer=w1762:i16)
                    n718 = To Word Integer(number=w1756) -> (16bit integer=w1761:i16)
                    n719 = Subtract(x=w1761, y=w1762) -> (x-y=w1760:i16)
                    n720 = Divide(x=w1758, y=3.413333333333333) -> (x/y=w1766:dbl)
                    n721 = Absolute Value(x=w1760) -> (abs(x)=w1759:i16)
                    n722 = Subtract(x=w1766, y=sgl 60.0) -> (x-y=w1764:dbl)
                    n723 = Greater?(x=w1759, y=u16 3) -> (0:w1755:bool)
                    n724 = Add(x=w1764, y=sgl 45.0) -> (x+y=w1754:dbl)
                    n725 = local write "Servo Moving - L"(w1755) -> ()
                    n726 = local write "Move Servo - L"(w1755) -> ()
                    n727 = local write "Current Angle\n - Left (internal)"(w1754) -> ()
                    n728 = shared-variable "RT myRIO Target - Overlord\\Localization_Variables_r0.lvlib\\Left Servo Angle_Current"(w1754) -> ()  [unwired: 1 in, 1 out]
                  }
                }
              }
              frame #2 {
                n729 = local read "Move Servo - L"() -> (w1771:bool)
                n730 = case shown="True" w1771 {
                  tunnel: w1774 -> [_ w1789]
                  tunnel: w1768 -> [_ w1776]
                  tunnel: [TRUE w1787] -> w1772
                  tunnel: w1773 -> [_ w1779]
                  tunnel: w1770 -> [_ w1778]
                  tunnel: w1769 -> [_ w1777]
                  frame False {
                    # "Only Send if Current Position is far enough"
                  }
                  frame True {
                    w1785 = 1
                    # "High Byte"
                    # "Low Byte"
                    n731 = Type Cast(type="", x=w1776) -> (*(type *) &x=w1786:string)
                    n732 = local write "Servo Moving - L"(TRUE) -> ()
                    n733 = String Subset(string=w1786, offset (0)=1, length (rest)=w1785) -> (substring=w1781:string)
                    n734 = String Subset(string=w1786, offset (0)=0, length (rest)=w1785) -> (substring=w1780:string)
                    n735 = while {
                      tunnel: w1789 -> [w1803]
                      tunnel: [w1795] -> w1787
                      tunnel: w1781 -> [w1799]
                      tunnel: w1780 -> [w1798]
                      tunnel: w1779 -> [w1792]
                      tunnel: w1778 -> [w1791]
                      tunnel: w1777 -> [w1790]
                      i -> [w1793]
                      stop <- w1794 stop-if-true
                      # "Attemp to Write Until\nMax Write Tx Attemps Limit"
                      n736 = call "MoveServo_R3.vi"("DIO Ref Out"=w1790, "VISA resource name out"=w1791, "GP - Low Byte"=w1799, "GP - High Byte"=w1798, "Servo ID"=w1803) -> ("Valid Checksum"=w1800:bool, "Error"=w1802:u64)  [unwired: 5 in]
                      n737 = Equal To 0?(x=w1802) -> (x = 0?=w1801:bool)
                      n738 = And(x=w1800, y=w1801) -> (x .and. y?=w1795:bool)
                      n739 = Increment(x=w1793) -> (x+1=w1797:i32)
                      n740 = Greater Or Equal?(x=w1797, y=w1792) -> (x >= y?=w1796:bool)
                      n741 = Or(x=w1795, y=w1796) -> (x .or. y?=w1794:bool)
                    }
                  }
                }
                n742 = case shown="True" w1772 {
                  frame False {
                  }
                  frame True {
                    # "Update Servo flag"
                    n743 = local write "Move Servo - L"(FALSE) -> ()
                  }
                }
              }
              frame #3 {
                n744 = call "Wait2"("Count(mSec)"="Servo Comm\nWait Time - (ms)") -> ()  [unwired: 1 out]
              }
              frame #4 {
                n745 = while {
                  tunnel: [w1827] -> w1813
                  tunnel: w1808 -> [w1826]
                  tunnel: [w1819] -> w1812
                  tunnel: w1814 -> [w1817]
                  tunnel: w1811 -> [w1816]
                  tunnel: w1810 -> [w1815]
                  i -> [w1818]
                  stop <- w1820 stop-if-true
                  # "Attemp to Read Until\nMax Read Tx Attemps Limit"
                  n746 = call "ReadServo_R3.vi"("DIO Ref In"=w1815, "VISA resource name out"=w1816, "Servo ID"=w1826) -> ("Error"=w1823:u8, "Valid Checksum"=w1824:bool, "Current Position"=w1827:u64)  [unwired: 6 in]
                  n747 = Increment(x=w1818) -> (x+1=w1821:i32)
                  n748 = Equal To 0?(x=w1823) -> (x = 0?=w1825:bool)
                  n749 = Greater Or Equal?(x=w1821, y=w1817) -> (x >= y?=w1822:bool)
                  n750 = And(x=w1824, y=w1825) -> (x .and. y?=w1819:bool)
                  n751 = Or(x=w1819, y=w1822) -> (x .or. y?=w1820:bool)
                }
              }
              frame #5 {
                n752 = local read "Servo Goal Position\n - Right"() -> (w1831:u16)
                n753 = case shown="True" w1833 {
                  tunnel: w1834 -> [_ w1838]
                  tunnel: w1831 -> [_ w1837]
                  frame False {
                    # "Don't update current position"
                  }
                  frame True {
                    # "Convert Received Position to Angle Relative to Robot"
                    # "45 DEG MOUNT OFFSET"
                    # "1024/300"
                    n754 = local write "Current R (10bit)"(w1838) -> ()
                    n755 = Divide(x=w1838, y=3.413333333333333) -> (x/y=w1847:dbl)
                    n756 = Subtract(x=w1847, y=sgl 60.0) -> (x-y=w1845:dbl)
                    n757 = Subtract(x=w1845, y=sgl 45.0) -> (x-y=w1835:dbl)
                    n758 = To Word Integer(number=w1837) -> (16bit integer=w1842:i16)
                    n759 = local write "Current Angle\n - Right (internal)"(w1835) -> ()
                    n760 = To Word Integer(number=w1838) -> (16bit integer=w1843:i16)
                    n761 = shared-variable "RT myRIO Target - Overlord\\Localization_Variables_r0.lvlib\\Right Servo Angle_Current"(w1835) -> ()  [unwired: 1 in, 1 out]
                    n762 = Subtract(x=w1842, y=w1843) -> (x-y=w1841:i16)
                    n763 = Absolute Value(x=w1841) -> (abs(x)=w1840:i16)
                    n764 = Greater?(x=w1840, y=u16 3) -> (0:w1836:bool)
                    n765 = local write "Servo Moving - R"(w1836) -> ()
                    n766 = local write "Move Servo - R"(w1836) -> ()
                  }
                }
              }
              frame #6 {
                n767 = local read "Move Servo - R"() -> (w1850:bool)
                n768 = case shown="True" w1850 {
                  tunnel: w1854 -> [_ w1859]
                  tunnel: w1856 -> [_ w1866]
                  tunnel: [TRUE w1867] -> w1851
                  tunnel: w1855 -> [_ w1862]
                  tunnel: w1853 -> [_ w1861]
                  tunnel: w1852 -> [_ w1860]
                  frame False {
                  }
                  frame True {
                    w1869 = 1
                    # "High Byte"
                    # "Low Byte"
                    n769 = Type Cast(type="", x=w1859) -> (*(type *) &x=w1868:string)
                    n770 = local write "Servo Moving - R"(TRUE) -> ()
                    n771 = String Subset(string=w1868, offset (0)=1, length (rest)=w1869) -> (substring=w1865:string)
                    n772 = String Subset(string=w1868, offset (0)=0, length (rest)=w1869) -> (substring=w1864:string)
                    n773 = while {
                      tunnel: [w1878] -> w1867
                      tunnel: w1866 -> [w1883]
                      tunnel: w1865 -> [w1882]
                      tunnel: w1864 -> [w1881]
                      tunnel: w1862 -> [w1876]
                      tunnel: w1861 -> [w1874]
                      tunnel: w1860 -> [w1873]
                      i -> [w1877]
                      stop <- w1875 stop-if-true
                      # "Attemp to Write Until\nMax Write Tx Attemps Limit"
                      n774 = call "MoveServo_R3.vi"("DIO Ref Out"=w1873, "VISA resource name out"=w1874, "GP - Low Byte"=w1882, "GP - High Byte"=w1881, "Servo ID"=w1883) -> ("Valid Checksum"=w1885:bool, "Error"=w1884:u64)  [unwired: 5 in]
                      n775 = Increment(x=w1877) -> (x+1=w1879:i32)
                      n776 = Greater Or Equal?(x=w1879, y=w1876) -> (x >= y?=w1880:bool)
                      n777 = Equal To 0?(x=w1884) -> (x = 0?=w1886:bool)
                      n778 = And(x=w1885, y=w1886) -> (x .and. y?=w1878:bool)
                      n779 = Or(x=w1878, y=w1880) -> (x .or. y?=w1875:bool)
                    }
                  }
                }
                n780 = case shown="True" w1851 {
                  frame False {
                  }
                  frame True {
                    # "Update Servo flag"
                    n781 = local write "Move Servo - R"(FALSE) -> ()
                  }
                }
              }
              frame #7 {
                n782 = call "Wait3"("Count(mSec)"=w1887) -> ()  [unwired: 1 out]
              }
              frame #8 {
                # "Increment Service Count"
                # "Update Compliance Slope\nEvery x loops"
                n783 = Equal?(x=w1891, y=u16 1000) -> (x = y?=w1900:bool)
                n784 = case shown="True" w1900 {
                  tunnel: w1896 -> [_ w1910]
                  tunnel: w1893 -> [_ w1909]
                  tunnel: w1892 -> [_ w1908]
                  tunnel: w1893 -> [_ w1907]
                  tunnel: w1892 -> [_ w1906]
                  tunnel: w1898 -> [_ w1905]
                  tunnel: w1897 -> [_ w1904]
                  tunnel: w1891 -> [w1901 _]
                  tunnel: [w1901 u16 0] -> w1899
                  tunnel: w1895 -> [_ w1902]
                  frame False {
                  }
                  frame True {
                    # "Reset Service\nCount"
                    n785 = flat-sequence {
                      tunnel: w1909 -> [w1915]
                      tunnel: w1908 -> [w1914]
                      tunnel: w1905 -> [w1916]
                      tunnel: [w1912] -> w1911
                      tunnel: w1910 -> [w1913]
                      tunnel: w1902 -> [w1912]
                      tunnel: w1904 -> [w1928]
                      tunnel: w1911 -> [w1927]
                      tunnel: w1910 -> [w1926]
                      tunnel: w1907 -> [w1925]
                      tunnel: w1906 -> [w1924]
                      frame #0 {
                        n786 = while {
                          tunnel: w1912 -> [w1923]
                          tunnel: w1915 -> [w1921]
                          tunnel: w1914 -> [w1920]
                          tunnel: w1916 -> [w1919]
                          tunnel: w1913 -> [w1918]
                          i -> [w1917]
                          stop <- w1922 stop-if-true
                          n787 = call "Set_Compliance_Slope_R2.vi"("Compliance Slope"=w1918, "DIO Ref Out"=w1920, "VISA resource name"=w1921, "Servo ID"=w1919) -> ()  [unwired: 6 in, 2 out]
                          n788 = Greater Or Equal?(x=w1917, y=w1923) -> (x >= y?=w1922:bool)
                        }
                      }
                      frame #1 {
                        n789 = while {
                          tunnel: w1927 -> [w1935]
                          tunnel: w1928 -> [w1933]
                          tunnel: w1925 -> [w1932]
                          tunnel: w1924 -> [w1931]
                          tunnel: w1926 -> [w1930]
                          i -> [w1929]
                          stop <- w1934 stop-if-true
                          n790 = call "Set_Compliance_Slope_R2.vi"("Compliance Slope"=w1930, "DIO Ref Out"=w1931, "VISA resource name"=w1932, "Servo ID"=w1933) -> ()  [unwired: 6 in, 2 out]
                          n791 = Greater Or Equal?(x=w1929, y=w1935) -> (x >= y?=w1934:bool)
                        }
                      }
                    }
                  }
                }
                n792 = Increment(x=w1899) -> (x+1=w1894:u16)
              }
            }
          }
        }
      }
    }
    frame #2 {
      n793 = VISA Close(VISA resource name=w1937) -> ()  [unwired: 1 in, 1 out]
      n794 = call <vilib>:"Close.vi"("DIO Ref In"=w1936) -> ()  [unwired: 10 in, 1 out]
    }
  }
